vi "W7XBolo2017_Flo.vi"(1 "FPGA VI Reference In":refnum<k20>) -> (0 "FPGA VI Reference Out":refnum<k20>)   [LabVIEW 2014]
uses:
  <vilib>/Platform/TimedLoop/XDataNode/timing_clust.ctl
  <vilib>/Platform/TimedLoop/XDataNode/nitl_modes.ctl
  <vilib>/Platform/TimedLoop/XDataNode/wakeup.ctl
  <vilib>/userdefined/High Color/nirio_resource_hc.ctl
  <vilib>/FPGAPlugInAG/PCI-7813R/niLvFpga_Open_PCI-7813R.vi
  <vilib>/Utility/error.llb/Error Cluster From Error Code.vi
  <vilib>/rvi/errors/niLvFpgaAdjustHostInterfaceError.vi
  <vilib>/Utility/file.llb/Read From Spreadsheet File (I64).vi
  <vilib>/rvi/interface/common/niFpgaWaitOnOcc.vi
  <vilib>/httpClient/POSTBuffer.vi
  <vilib>/FPGAPlugInAG/PCI-7813R/niLvFpga_Close_PCI-7813R.vi
  <vilib>/Platform/TimedLoop/XDataNode/XDataNode.xnode
  <vilib>/rvi/interface/nirviOpenFPGA/nirviOpenFPGA.xnode
  FPGA Bitfiles/W7XBolo2017_FPGATarget_FlorianDefault.lvbitx
  f_main_2014.vi
  <vilib>/rvi/interface/nirviReadWriteControl/nirviReadWriteControl.xnode
  <vilib>/rvi/interface/nirviMethod/nirviMethod.xnode
  <vilib>/rvi/interface/nirviCloseFPGA/nirviCloseFPGA.xnode
  <vilib>/Platform/TimedLoop/XDataNode/XDNodeRunTimeDep.lvlib
  <vilib>/Analysis/NI_AALBase.lvlib
  <vilib>/httpClient/LabVIEWHTTPClient.lvlib
  NiFpgaLv.dll
  <vilib>/FPGAPlugInAG/PCI-7813R/niLvFpga_AcknowledgeIrq_PCI-7813R.vi
  <vilib>/FPGAPlugInAG/PCI-7813R/niLvFpga_ConfigureFifo_PCI-7813R.vi
  <vilib>/rvi/errors/niLvFpgaMergeErrorWithErrorCode.vi
panel:
  out "DAQ Timer":dbl
  in  "chanDescs":T1(array[cluster])=[{"name"="HBCm_U30_01", "active"=1, "physicalQuantity"={"type"="A"}}, {"name"="HBCm_U30_02", "active"=1, "physicalQuantity"={"type"="A"}}, {"name"="HBCm_U30_03", "active"=1, "physicalQuantity"={"type"="A"}}, {"name"="HBCm_U30_04", "active"=1, "physicalQuantity"={"type"="A"}}, {"name"="HBCm_U30_05", "active"=1, "physicalQuantity"={"type"="A"}}, {"name"="HBCm_U30_06", "active"=1, "physicalQuantity"={"type"="A"}}, {"name"="HBCm_U30_07", "active"=1, "physicalQuantity"={"type"="A"}}, {"name"="HBCm_U30_08", "active"=1, "physicalQuantity"={"type"="A"}}, {"name"="HBCm_U30_09", "active"=1, "physicalQuantity"={"type"="A"}}, {"name"="HBCm_U30_10", "active"=1, "physicalQuantity"={"type"="A"}}, {"name"="HBCm_U30_11", "active"=1, "physicalQuantity"={"type"="A"}}, {"name"="HBCm_U30_12", "active"=1, "physicalQuantity"={"type"="A"}}, {"name"="HBCm_U30_013", "active"=1, "physicalQuantity"={"type"="A"}}, {"name"="HBCm_U30_14", "active"=1, "physicalQuantity"={"type"="A"}}, {"name"="HBCm_U30_15", "active"=1, "physicalQuantity"={"type"="A"}}, {"name"="HBCm_U30_16", "active"=1, "physicalQuantity"={"type"="A"}}, {"name"="HBCm_U30_17", "active"=1, "physicalQuantity"={"type"="A"}}, {"name"="HBCm_U30_18", "active"=1, "physicalQuantity"={"type"="A"}}, {"name"="HBCm_U30_19", "active"=1, "physicalQuantity"={"type"="A"}}, {"name"="HBCm_U30_20", "active"=1, "physicalQuantity"={"type"="A"}}, {"name"="HBCm_U30_21", "active"=1, "physicalQuantity"={"type"="A"}}, {"name"="HBCm_U30_22", "active"=1, "physicalQuantity"={"type"="A"}}, {"name"="HBCm_U30_23", "active"=1, "physicalQuantity"={"type"="A"}}, {"name"="HBCm_U30_24", "active"=1, "physicalQuantity"={"type"="A"}}, {"name"="HBCm_U30_25", "active"=1, "physicalQuantity"={"type"="A"}}, {"name"="HBCm_U30_26", "active"=1, "physicalQuantity"={"type"="A"}}, {"name"="HBCm_U30_27", "active"=1, "physicalQuantity"={"type"="A"}}, {"name"="HBCm_U30_28", "active"=1, "physicalQuantity"={"type"="A"}}, {"name"="HBCm_U30_29", "active"=1, "physicalQuantity"={"type"="A"}}, {"name"="HBCm_U30_30", "active"=1, "physicalQuantity"={"type"="A"}}, {"name"="HBCm_U30_31", "active"=1, "physicalQuantity"={"type"="A"}}, {"name"="HBCm_U30_32", "active"=1, "physicalQuantity"={"type"="A"}}, {"name"="VBCm_V21_01", "active"=1, "physicalQuantity"={"type"="A"}}, {"name"="VBCm_V21_02", "active"=1, "physicalQuantity"={"type"="A"}}, {"name"="VBCm_V21_03", "active"=1, "physicalQuantity"={"type"="A"}}, {"name"="VBCm_V21_04", "active"=1, "physicalQuantity"={"type"="A"}}, {"name"="VBCm_V21_05", "active"=1, "physicalQuantity"={"type"="A"}}, {"name"="VBCm_V21_06", "active"=1, "physicalQuantity"={"type"="A"}}, {"name"="VBCm_V21_07", "active"=1, "physicalQuantity"={"type"="A"}}, {"name"="VBCm_V21_08", "active"=1, "physicalQuantity"={"type"="A"}}, {"name"="VBCm_V21_09", "active"=1, "physicalQuantity"={"type"="A"}}, {"name"="VBCm_V21_10", "active"=1, "physicalQuantity"={"type"="A"}}, {"name"="VBCm_V21_11", "active"=1, "physicalQuantity"={"type"="A"}}, {"name"="VBCm_V21_12", "active"=1, "physicalQuantity"={"type"="A"}}, {"name"="VBCm_V21_13", "active"=1, "physicalQuantity"={"type"="A"}}, {"name"="VBCm_V21_14", "active"=1, "physicalQuantity"={"type"="A"}}, {"name"="VBCm_V21_15", "active"=1, "physicalQuantity"={"type"="A"}}, {"name"="VBCm_V21_16", "active"=1, "physicalQuantity"={"type"="A"}}, {"name"="VBCm_V21_17", "active"=1, "physicalQuantity"={"type"="A"}}, {"name"="VBCm_V21_18", "active"=1, "physicalQuantity"={"type"="A"}}, {"name"="VBCm_V21_19", "active"=1, "physicalQuantity"={"type"="A"}}, {"name"="VBCm_V21_20", "active"=1, "physicalQuantity"={"type"="A"}}, {"name"="VBCm_V21_21", "active"=1, "physicalQuantity"={"type"="A"}}, {"name"="VBCm_V21_22", "active"=1, "physicalQuantity"={"type"="A"}}, {"name"="VBCm_V21_23", "active"=1, "physicalQuantity"={"type"="A"}}, {"name"="VBCm_V21_24", "active"=1, "physicalQuantity"={"type"="A"}}, {"name"="VBCm_V21_25", "active"=1, "physicalQuantity"={"type"="A"}}, {"name"="VBCm_V21_26", "active"=1, "physicalQuantity"={"type"="A"}}, {"name"="VBCm_V21_27", "active"=1, "physicalQuantity"={"type"="A"}}, {"name"="VBCm_V21_28", "active"=1, "physicalQuantity"={"type"="A"}}, {"name"="VBCm_V21_29", "active"=1, "physicalQuantity"={"type"="A"}}, {"name"="VBCm_V21_30", "active"=1, "physicalQuantity"={"type"="A"}}, {"name"="VBCm_V21_31", "active"=1, "physicalQuantity"={"type"="A"}}, {"name"="VBCm_V21_32", "active"=1, "physicalQuantity"={"type"="A"}}, {"name"="VBCm_V21_33", "active"=1, "physicalQuantity"={"type"="A"}}, {"name"="VBCm_V21_34", "active"=1, "physicalQuantity"={"type"="A"}}, {"name"="VBCm_V21_35", "active"=1, "physicalQuantity"={"type"="A"}}, {"name"="VBCm_V21_36", "active"=1, "physicalQuantity"={"type"="A"}}, {"name"="VBCm_V21_37", "active"=1, "physicalQuantity"={"type"="A"}}, {"name"="VBCm_V21_38", "active"=1, "physicalQuantity"={"type"="A"}}, {"name"="VBCm_V21_39", "active"=1, "physicalQuantity"={"type"="A"}}, {"name"="VBCm_V21_40", "active"=1, "physicalQuantity"={"type"="A"}}, {"name"="VBCs_V21_01", "active"=1, "physicalQuantity"={"type"="A"}}, {"name"="VBCs_V21_02", "active"=1, "physicalQuantity"={"type"="A"}}, {"name"="VBCs_V21_03", "active"=1, "physicalQuantity"={"type"="A"}}, {"name"="VBCs_V21_04", "active"=1, "physicalQuantity"={"type"="A"}}, {"name"="VBCs_V21_05", "active"=1, "physicalQuantity"={"type"="A"}}, {"name"="VBCs_V21_06", "active"=1, "physicalQuantity"={"type"="A"}}, {"name"="VBCs_V21_07", "active"=1, "physicalQuantity"={"type"="A"}}, {"name"="VBCs_V21_08", "active"=1, "physicalQuantity"={"type"="A"}}, {"name"="HBCs_U30_01", "active"=1, "physicalQuantity"={"type"="A"}}, {"name"="HBCs_U30_02", "active"=1, "physicalQuantity"={"type"="A"}}, {"name"="HBCs_U30_03", "active"=1, "physicalQuantity"={"type"="A"}}, {"name"="HBCs_U30_04", "active"=1, "physicalQuantity"={"type"="A"}}, {"name"="HBCs_U30_05", "active"=1, "physicalQuantity"={"type"="A"}}, {"name"="HBCs_U30_06", "active"=1, "physicalQuantity"={"type"="A"}}, {"name"="HBCs_U30_07", "active"=1, "physicalQuantity"={"type"="A"}}, {"name"="HBCs_U30_08", "active"=1, "physicalQuantity"={"type"="A"}}, {"name"="HBCs_U30_09", "active"=1, "physicalQuantity"={"type"="A"}}, {"name"="HBCs_U30_10", "active"=1, "physicalQuantity"={"type"="A"}}, {"name"="HBCs_U30_11", "active"=1, "physicalQuantity"={"type"="A"}}, {"name"="HBCs_U30_12", "active"=1, "physicalQuantity"={"type"="A"}}, {"name"="HBCs_U30_13", "active"=1, "physicalQuantity"={"type"="A"}}, {"name"="HBCs_U30_14", "active"=1, "physicalQuantity"={"type"="A"}}, {"name"="HBCs_U30_15", "active"=1, "physicalQuantity"={"type"="A"}}, {"name"="HBCs_U30_16", "active"=1, "physicalQuantity"={"type"="A"}}]
  in  "Tab Control 7":T2(tab)
  in  "FreqSelRing":u16(ring) items=["0.8 ms", "1.6 ms", "3.2 ms", "6.4 ms", "12.8 ms", "19.2 ms"]
  in  "SecondFilter":bool=TRUE
  out "SampleTime":sgl=0.0004
  in  "Global or Individual\nDAC Settings loaded \nfrom File":bool=TRUE caption="Range?"
  in  "DAC Range Setting":u8(knob)=3 scale=0.0..3.0
  in  "No. of Samples:":u32=10000
  out "Measured Time \nfor DAQ [ms] \nShould ~ correspond to\nSampleTime * Samples":u32=8048
  in  "Trigger Source":i32(slide)=1 scale=0.0..2.0
  in  "Set Manual Time [ns]":i64=1503619200000000000
  out "Presamples \n(If -1, then no trigger detected)":i32
  out "DAQ wait time (should be = TWT":i32=-1
  out "Countdown Time":u32
  out "Calibration Time":u32
  out "Total wait time (TWT)\nTypically 59 s":u32
  in  "Pre-start time (ms) of DAQ \nTypically set to 1000 ms":i32=1000
  out "Fixed T-60sec before T1 = T0":i32=60000
  in  "Wait-Time until Trigger\npublished on CODA\ntypically 10 s":u32=10000
  in  "Tau00":dbl[](array[numeric])
  in  "Kappa00":dbl[](array[numeric])
  in  "RB000":dbl[](array[numeric])
  in  "Switch to fixed \nCalibration Values":bool
  in  "Clear all Values \nfrom Beginning":bool
  in  "Cancel Button":bool
  out "Actual Depth":u32=256
  out "T-Start [for Display)\nShould be -1 [s]":sgl=-1.0
  in  "Trigger No Choice\nfrom MDS+ Website\n0 for old\n1 during OP":i32
  out "body chanDesc":string="Test/raw/W7X/QSB_Bolometry/File_PARLOG/ created."
  out "headers chanDesc":string="HTTP/1.1 201 Created\r\nServer: Apache-Coyote/1.1\r\nLocation: http://archive-webapi.ipp-hgw.mpg.de/Test/raw/W7X/QSB_Bolometry/File_PARLOG/\r\nContent-Type: text/plain\r\nTransfer-Encoding: chunked\r\nDate: Wed, 15 Jul 2015 13:52:20 GMT\r\n\r\n"
  out "parms error out":errorcluster
  in  "Tab Control":T3(tab)
  in  "Tab Control 4":enum32{"1 to 64", "65 to 128"}(tab)
  out "Raw 33-64":T4={"Channels 33 - 40"={"tstart"=-1.0, "FPGSampleTime"=0.0007999999797903001, array8x10000[80000 elements]}, "Channels 41 - 48"={"tstart"=-1.0, "FPGSampleTime"=0.0007999999797903001, array8x10000[80000 elements]}, "Channels 49 - 56"={"tstart"=-1.0, "FPGSampleTime"=0.0007999999797903001, array8x10000[80000 elements]}, "Channels 57 - 64"={"tstart"=-1.0, "FPGSampleTime"=0.0007999999797903001, array8x10000[80000 elements]}}
  out "Raw 1-32":T5={"Channels 1- 8"={"tstart"=-1.0, "FPGSampleTime"=0.0007999999797903001, array8x10000[80000 elements]}, "Channels 9 - 16"={"tstart"=-1.0, "FPGSampleTime"=0.0007999999797903001, array8x10000[80000 elements]}, "Channels 17 - 24"={"tstart"=-1.0, "FPGSampleTime"=0.0007999999797903001, array8x10000[80000 elements]}, "Channels 25 - 32"={"tstart"=-1.0, "FPGSampleTime"=0.0007999999797903001, array8x10000[80000 elements]}}
  out "Raw 97 - 128":T6
  out "Raw 65 - 97":T7={"Channels 65 - 71"={"tstart"=-1.0, "FPGSampleTime"=0.0007999999797903001, array8x10000[80000 elements]}, "Channels 73 - 80"={"tstart"=0.0, "FPGSampleTime"=0.0, []}, "Channels 81 - 88"={"tstart"=0.0, "FPGSampleTime"=0.0, []}, "Channels 89- 96"={"tstart"=0.0, "FPGSampleTime"=0.0, []}}
  in  "Tab Control 6":enum32{"1 to 64", "65 to 128"}(tab)=enum."65 to 128"
  out "Pow 33-64":T4
  out "Pow 1-32":T5={"Channels 1- 8"={"tstart"=-1.0, "FPGSampleTime"=0.0007999999797903001, array8x10000[80000 elements]}, "Channels 9 - 16"={"tstart"=-1.0, "FPGSampleTime"=0.0007999999797903001, array8x10000[80000 elements]}, "Channels 17 - 24"={"tstart"=0.0, "FPGSampleTime"=0.0, []}, "Channels 25 - 32"={"tstart"=0.0, "FPGSampleTime"=0.0, []}}
  out "Pow 97 - 128":T6
  out "Pow 65 - 96":T7={"Channels 65 - 71"={"tstart"=-1.0, "FPGSampleTime"=0.0007999999797903001, array8x10000[80000 elements]}, "Channels 73 - 80"={"tstart"=0.0, "FPGSampleTime"=0.0, []}, "Channels 81 - 88"={"tstart"=0.0, "FPGSampleTime"=0.0, []}, "Channels 89- 96"={"tstart"=0.0, "FPGSampleTime"=0.0, []}}
  out "RangeIndex":u8[](array[numeric])
  out "DACbits 2":u16[](array[numeric])
  in  "file path (dialog if empty)":path=path "C:/W7-X-DAQ-Data/_DAQ_Ranges.txt"
  in  "Tab Control 2":T8(tab)
  out "Offset 1-32":T5
  out "Offset 33-64":T4
  out "Offset 65 - 96":T7
  out "Offset 97 - 128":T6
  out "Mean (mV)":dbl[](array[numeric]) format="%10.6f"
  out "Peak to Peak \n      (microV)":dbl[](array[numeric]) format="%10.6f"
  out "StandardDeviation\n        (microV)":dbl[](array[numeric]) format="%10.7f"
  out "RefStatus 65-96":bool[](array[boolean])
  out "RefStatus 33-64":bool[](array[boolean])
  out "RefStatus 1-32":bool[](array[boolean])
  out "RefStatus 97-128":bool[](array[boolean])
  out "MessStatus 1-32":bool[](array[boolean])
  out "MessStatus 33-64":bool[](array[boolean])
  out "MessStatus 97-128":bool[](array[boolean])
  out "MessStatus 65-96":bool[](array[boolean])
  in  "Tab Control 5":T9(tab)
  out "MessCal 17-32":T10
  out "MessCal 1-16":T11
  out "MessCal 49 - 64":T12
  out "MessCal 33 - 49":T13
  out "MessCal 81 - 96":T14
  out "MessCal 65 - 80":T15
  out "MessCal 113 - 128":T16
  out "MessCal 97 - 112":T17
  out "RMESS":dbl[](array[numeric])
  out "KappaM":dbl[](array[numeric]) format="%10.4e"
  out "TauM":dbl[](array[numeric]) format="%10.4f"
  in  "Tab Control 3":T9(tab)=enum."97 to 128"
  out "RefCal 17-32":T10
  out "RefCal 1-16":T11
  out "RefCal 49 - 64":T12
  out "RefCal 33 - 48":T13
  out "RefCal 65 - 80":T15
  out "RefCal 81 - 96":T14
  out "RefCal 113 - 128":T16
  out "RefCal 97 - 112":T17
  out "TauR":dbl[](array[numeric]) caption="TauM" format="%10.4f"
  out "KappaR":dbl[](array[numeric]) format="%10.4e"
  out "RREF":dbl[](array[numeric])
  out "Parlog error out":errorcluster
  out "Parlog error out  2":errorcluster
  out "Parlog error out  3":errorcluster
  out "error out":errorcluster
  out "Timed Out 2":bool
  out "Fehler":bool
  out "Fehler READ U+P":bool
  out "FilterTimeOut":bool
  out "result":bool
  out "chanDescs 2":T1(array[cluster])=[{"name"="HBCm_U30_01", "active"=1, "physicalQuantity"={"type"="A"}}, {"name"="HBCm_U30_02", "active"=1, "physicalQuantity"={"type"="A"}}, {"name"="HBCm_U30_03", "active"=1, "physicalQuantity"={"type"="A"}}, {"name"="HBCm_U30_04", "active"=1, "physicalQuantity"={"type"="A"}}, {"name"="HBCm_U30_05", "active"=1, "physicalQuantity"={"type"="A"}}, {"name"="HBCm_U30_06", "active"=1, "physicalQuantity"={"type"="A"}}, {"name"="HBCm_U30_07", "active"=1, "physicalQuantity"={"type"="A"}}, {"name"="HBCm_U30_08", "active"=1, "physicalQuantity"={"type"="A"}}, {"name"="HBCm_U30_09", "active"=1, "physicalQuantity"={"type"="A"}}, {"name"="HBCm_U30_10", "active"=1, "physicalQuantity"={"type"="A"}}, {"name"="HBCm_U30_11", "active"=1, "physicalQuantity"={"type"="A"}}, {"name"="HBCm_U30_12", "active"=1, "physicalQuantity"={"type"="A"}}, {"name"="HBCm_U30_13", "active"=1, "physicalQuantity"={"type"="A"}}, {"name"="HBCm_U30_14", "active"=1, "physicalQuantity"={"type"="A"}}, {"name"="HBCm_U30_15", "active"=1, "physicalQuantity"={"type"="A"}}, {"name"="HBCm_U30_16", "active"=1, "physicalQuantity"={"type"="A"}}, {"name"="HBCm_U30_17", "active"=1, "physicalQuantity"={"type"="A"}}, {"name"="HBCm_U30_18", "active"=1, "physicalQuantity"={"type"="A"}}, {"name"="HBCm_U30_19", "active"=1, "physicalQuantity"={"type"="A"}}, {"name"="HBCm_U30_20", "active"=1, "physicalQuantity"={"type"="A"}}, {"name"="HBCm_U30_21", "active"=1, "physicalQuantity"={"type"="A"}}, {"name"="HBCm_U30_22", "active"=1, "physicalQuantity"={"type"="A"}}, {"name"="HBCm_U30_23", "active"=1, "physicalQuantity"={"type"="A"}}, {"name"="HBCm_U30_24", "active"=1, "physicalQuantity"={"type"="A"}}, {"name"="HBCm_U30_25", "active"=1, "physicalQuantity"={"type"="A"}}, {"name"="HBCm_U30_26", "active"=1, "physicalQuantity"={"type"="A"}}, {"name"="HBCm_U30_27", "active"=1, "physicalQuantity"={"type"="A"}}, {"name"="HBCm_U30_28", "active"=1, "physicalQuantity"={"type"="A"}}, {"name"="HBCm_U30_29", "active"=1, "physicalQuantity"={"type"="A"}}, {"name"="HBCm_U30_30", "active"=1, "physicalQuantity"={"type"="A"}}, {"name"="HBCm_U30_31", "active"=1, "physicalQuantity"={"type"="A"}}, {"name"="HBCm_U30_32", "active"=1, "physicalQuantity"={"type"="A"}}, {"name"="VBCm_V21_01", "active"=1, "physicalQuantity"={"type"="A"}}, {"name"="VBCm_V21_02", "active"=1, "physicalQuantity"={"type"="A"}}, {"name"="VBCm_V21_03", "active"=1, "physicalQuantity"={"type"="A"}}, {"name"="VBCm_V21_04", "active"=1, "physicalQuantity"={"type"="A"}}, {"name"="VBCm_V21_05", "active"=1, "physicalQuantity"={"type"="A"}}, {"name"="VBCm_V21_06", "active"=1, "physicalQuantity"={"type"="A"}}, {"name"="VBCm_V21_07", "active"=1, "physicalQuantity"={"type"="A"}}, {"name"="VBCm_V21_08", "active"=1, "physicalQuantity"={"type"="A"}}, {"name"="VBCm_V21_09", "active"=1, "physicalQuantity"={"type"="A"}}, {"name"="VBCm_V21_10", "active"=1, "physicalQuantity"={"type"="A"}}, {"name"="VBCm_V21_11", "active"=1, "physicalQuantity"={"type"="A"}}, {"name"="VBCm_V21_12", "active"=1, "physicalQuantity"={"type"="A"}}, {"name"="VBCm_V21_13", "active"=1, "physicalQuantity"={"type"="A"}}, {"name"="VBCm_V21_14", "active"=1, "physicalQuantity"={"type"="A"}}, {"name"="VBCm_V21_15", "active"=1, "physicalQuantity"={"type"="A"}}, {"name"="VBCm_V21_16", "active"=1, "physicalQuantity"={"type"="A"}}, {"name"="VBCm_V21_17", "active"=1, "physicalQuantity"={"type"="A"}}, {"name"="VBCm_V21_18", "active"=1, "physicalQuantity"={"type"="A"}}, {"name"="VBCm_V21_19", "active"=1, "physicalQuantity"={"type"="A"}}, {"name"="VBCm_V21_20", "active"=1, "physicalQuantity"={"type"="A"}}, {"name"="VBCm_V21_21", "active"=1, "physicalQuantity"={"type"="A"}}, {"name"="VBCm_V21_22", "active"=1, "physicalQuantity"={"type"="A"}}, {"name"="VBCm_V21_23", "active"=1, "physicalQuantity"={"type"="A"}}, {"name"="VBCm_V21_24", "active"=1, "physicalQuantity"={"type"="A"}}, {"name"="VBCm_V21_25", "active"=1, "physicalQuantity"={"type"="A"}}, {"name"="VBCm_V21_26", "active"=1, "physicalQuantity"={"type"="A"}}, {"name"="VBCm_V21_27", "active"=1, "physicalQuantity"={"type"="A"}}, {"name"="VBCm_V21_28", "active"=1, "physicalQuantity"={"type"="A"}}, {"name"="VBCm_V21_29", "active"=1, "physicalQuantity"={"type"="A"}}, {"name"="VBCm_V21_30", "active"=1, "physicalQuantity"={"type"="A"}}, {"name"="VBCm_V21_31", "active"=1, "physicalQuantity"={"type"="A"}}, {"name"="VBCm_V21_32", "active"=1, "physicalQuantity"={"type"="A"}}, {"name"="VBCm_V21_33", "active"=1, "physicalQuantity"={"type"="A"}}, {"name"="VBCm_V21_34", "active"=1, "physicalQuantity"={"type"="A"}}, {"name"="VBCm_V21_35", "active"=1, "physicalQuantity"={"type"="A"}}, {"name"="VBCm_V21_36", "active"=1, "physicalQuantity"={"type"="A"}}, {"name"="VBCm_V21_37", "active"=1, "physicalQuantity"={"type"="A"}}, {"name"="VBCm_V21_38", "active"=1, "physicalQuantity"={"type"="A"}}, {"name"="VBCm_V21_39", "active"=1, "physicalQuantity"={"type"="A"}}, {"name"="VBCm_V21_40", "active"=1, "physicalQuantity"={"type"="A"}}, {"name"="VBCs_V21_01", "active"=1, "physicalQuantity"={"type"="A"}}, {"name"="VBCs_V21_02", "active"=1, "physicalQuantity"={"type"="A"}}, {"name"="VBCs_V21_03", "active"=1, "physicalQuantity"={"type"="A"}}, {"name"="VBCs_V21_04", "active"=1, "physicalQuantity"={"type"="A"}}, {"name"="VBCs_V21_05", "active"=1, "physicalQuantity"={"type"="A"}}, {"name"="VBCs_V21_06", "active"=1, "physicalQuantity"={"type"="A"}}, {"name"="VBCs_V21_07", "active"=1, "physicalQuantity"={"type"="A"}}, {"name"="VBCs_V21_08", "active"=1, "physicalQuantity"={"type"="A"}}, {"name"="HBCs_U30_01", "active"=1, "physicalQuantity"={"type"="A"}}, {"name"="HBCs_U30_02", "active"=1, "physicalQuantity"={"type"="A"}}, {"name"="HBCs_U30_03", "active"=1, "physicalQuantity"={"type"="A"}}, {"name"="HBCs_U30_04", "active"=1, "physicalQuantity"={"type"="A"}}, {"name"="HBCs_U30_05", "active"=1, "physicalQuantity"={"type"="A"}}, {"name"="HBCs_U30_06", "active"=1, "physicalQuantity"={"type"="A"}}, {"name"="HBCs_U30_07", "active"=1, "physicalQuantity"={"type"="A"}}, {"name"="HBCs_U30_08", "active"=1, "physicalQuantity"={"type"="A"}}, {"name"="HBCs_U30_09", "active"=1, "physicalQuantity"={"type"="A"}}, {"name"="HBCs_U30_10", "active"=1, "physicalQuantity"={"type"="A"}}, {"name"="HBCs_U30_11", "active"=1, "physicalQuantity"={"type"="A"}}, {"name"="HBCs_U30_12", "active"=1, "physicalQuantity"={"type"="A"}}, {"name"="HBCs_U30_13", "active"=1, "physicalQuantity"={"type"="A"}}, {"name"="HBCs_U30_14", "active"=1, "physicalQuantity"={"type"="A"}}, {"name"="HBCs_U30_15", "active"=1, "physicalQuantity"={"type"="A"}}, {"name"="HBCs_U30_16", "active"=1, "physicalQuantity"={"type"="A"}}, {"name"="Test96", "active"=1, "physicalQuantity"={"type"="A"}}, {"name"="Test97", "active"=0, "physicalQuantity"={"type"=""}}]
  out "error out Cal":errorcluster
  in  "stop":bool
  out "Acquired Samples:":u32(slide) scale=-1.0..10000.0
  out "state":string="Wait for Start"
  # "Largest Offset ~ 20 mV\n40 mV Range should work \nfor all channels"
  # "Sample Rate Settings"
  # "FilterSelection"
  # "Set manual time above"
  # "Get last trigger fr om \nhttp://sv-coda-wsvc-3/last_trigger"
  # "Get UTC Time not working"
  # "WENDELSTEIN - 7-X Bolometer DAQ System"
  # "ver 2017"
  # "If individual Range DAC Setting is selected, \nthe gain Range is loaded from following file:"
  # "DAC Range shown for check:"
types:
  T1 = cluster{"name":string, "active":i32, "physicalQuantity":cluster{"type":string}}[]
  T2 = enum32{"DAQ Settings", "Trigger Selection", "Fixed Calib Values", "Experimental"}
  T3 = enum32{"Raw", "Power", "Indiviudal Range Settings", "Offsets", "Status", "CalibMess", "CalibRef", "Errors and others"}
  T4 = cluster{"Channels 33 - 40":cluster{"tstart":dbl, "FPGSampleTime":dbl, dbl[][]}, "Channels 41 - 48":cluster{"tstart":dbl, "FPGSampleTime":dbl, dbl[][]}, "Channels 49 - 56":cluster{"tstart":dbl, "FPGSampleTime":dbl, dbl[][]}, "Channels 57 - 64":cluster{"tstart":dbl, "FPGSampleTime":dbl, dbl[][]}}
  T5 = cluster{"Channels 1- 8":cluster{"tstart":dbl, "FPGSampleTime":dbl, dbl[][]}, "Channels 9 - 16":cluster{"tstart":dbl, "FPGSampleTime":dbl, dbl[][]}, "Channels 17 - 24":cluster{"tstart":dbl, "FPGSampleTime":dbl, dbl[][]}, "Channels 25 - 32":cluster{"tstart":dbl, "FPGSampleTime":dbl, dbl[][]}}
  T6 = cluster{"Channels 97 - 104":cluster{"tstart":dbl, "FPGSampleTime":dbl, dbl[][]}, "Channels 105 - 112":cluster{"tstart":dbl, "FPGSampleTime":dbl, dbl[][]}, "Channels 113 - 120":cluster{"tstart":dbl, "FPGSampleTime":dbl, dbl[][]}, "Channels 121 - 128":cluster{"tstart":dbl, "FPGSampleTime":dbl, dbl[][]}}
  T7 = cluster{"Channels 65 - 71":cluster{"tstart":dbl, "FPGSampleTime":dbl, dbl[][]}, "Channels 73 - 80":cluster{"tstart":dbl, "FPGSampleTime":dbl, dbl[][]}, "Channels 81 - 88":cluster{"tstart":dbl, "FPGSampleTime":dbl, dbl[][]}, "Channels 89- 96":cluster{"tstart":dbl, "FPGSampleTime":dbl, dbl[][]}}
  T8 = enum32{"1 to 32", "33 to 64", "65 to 96", "97 to128"}
  T9 = enum32{"1 to 32", "33 to 64", "65 to 96", "97 to 128"}
  T10 = cluster{"Channels 17 - 20":cluster{"tstart":sgl, "dt":sgl, "OutArray":dbl[][]}, "Channels 21 - 24":cluster{"tstart":sgl, "dt":sgl, "OutArray":dbl[][]}, "Channels 25 - 28":cluster{"tstart":sgl, "dt":sgl, "OutArray":dbl[][]}, "Channels 29 - 32":cluster{"tstart":sgl, "dt":sgl, "OutArray":dbl[][]}}
  T11 = cluster{"Channels 1- 4":cluster{"tstart":sgl, "dt":sgl, "OutArray":dbl[][]}, "Channels 5 - 8":cluster{"tstart":sgl, "dt":sgl, "OutArray":dbl[][]}, "Channels 9 - 12":cluster{"tstart":sgl, "dt":sgl, "OutArray":dbl[][]}, "Channels 13 - 16":cluster{"tstart":sgl, "dt":sgl, "OutArray":dbl[][]}}
  T12 = cluster{"Channels 49 - 52":cluster{"tstart":sgl, "dt":sgl, "OutArray":dbl[][]}, "Channels 53 - 56":cluster{"tstart":sgl, "dt":sgl, "OutArray":dbl[][]}, "Channels 57 - 60":cluster{"tstart":sgl, "dt":sgl, "OutArray":dbl[][]}, "Channels 61 - 64":cluster{"tstart":sgl, "dt":sgl, "OutArray":dbl[][]}}
  T13 = cluster{"Channels 33 - 36":cluster{"tstart":sgl, "dt":sgl, "OutArray":dbl[][]}, "Channels 37 - 40":cluster{"tstart":sgl, "dt":sgl, "OutArray":dbl[][]}, "Channels 41 - 44":cluster{"tstart":sgl, "dt":sgl, "OutArray":dbl[][]}, "Channels 45 - 48":cluster{"tstart":sgl, "dt":sgl, "OutArray":dbl[][]}}
  T14 = cluster{"Channels 81 - 84":cluster{"tstart":sgl, "dt":sgl, "OutArray":dbl[][]}, "Channels 85 - 88":cluster{"tstart":sgl, "dt":sgl, "OutArray":dbl[][]}, "Channels 89 - 92":cluster{"tstart":sgl, "dt":sgl, "OutArray":dbl[][]}, "Channels 93 - 96":cluster{"tstart":sgl, "dt":sgl, "OutArray":dbl[][]}}
  T15 = cluster{"Channels 65 - 68":cluster{"tstart":sgl, "dt":sgl, "OutArray":dbl[][]}, "Channels 69 - 72":cluster{"tstart":sgl, "dt":sgl, "OutArray":dbl[][]}, "Channels 73 - 76":cluster{"tstart":sgl, "dt":sgl, "OutArray":dbl[][]}, "Channels 77 - 80":cluster{"tstart":sgl, "dt":sgl, "OutArray":dbl[][]}}
  T16 = cluster{"Channels 113 - 116":cluster{"tstart":sgl, "dt":sgl, "OutArray":dbl[][]}, "Channels 117 - 120":cluster{"tstart":sgl, "dt":sgl, "OutArray":dbl[][]}, "Channels 121 - 124":cluster{"tstart":sgl, "dt":sgl, "OutArray":dbl[][]}, "Channels 125 - 128":cluster{"tstart":sgl, "dt":sgl, "OutArray":dbl[][]}}
  T17 = cluster{"Channels 97 - 100":cluster{"tstart":sgl, "dt":sgl, "OutArray":dbl[][]}, "Channels 101 - 104":cluster{"tstart":sgl, "dt":sgl, "OutArray":dbl[][]}, "Channels 104 - 108":cluster{"tstart":sgl, "dt":sgl, "OutArray":dbl[][]}, "Channels 109 - 112":cluster{"tstart":sgl, "dt":sgl, "OutArray":dbl[][]}}
  T18 = cluster{"Nchannel":i16, "ADCbits":i16, "BridgeVoltage (V)":sgl, "ExptSampleFrequency (Hz)":sgl, "CalibSampleFrequency (Hz)":sgl, "CalStep1 (V)":string, "CalStep2 (V)":string, "detector":string}[]
  T19 = cluster{"chanDescs":cluster{"name":string, "active":i32}[]}[]
  T20 = cluster{"tstart":sgl, "dt":sgl, "OutArray":dbl[][]}
  T21 = cluster{"Channels 9 - 12":cluster{"tstart":sgl, "dt":sgl, "OutArray":dbl[][]}, "Channels 9 - 12":cluster{"tstart":sgl, "dt":sgl, "OutArray":dbl[][]}, "Channels 9 - 12":cluster{"tstart":sgl, "dt":sgl, "OutArray":dbl[][]}, "Channels 9 - 12":cluster{"tstart":sgl, "dt":sgl, "OutArray":dbl[][]}}
  T22 = typedef "nirio_resource_hc.ctl" = tag
  T23 = typedef "XDNodeRunTimeDep.lvlib/timing_clust.ctl" = cluster{"Expected End [f-1]":u64, "Actual End [f-1]":u64, "Finished Late? [f-1]":bool, "Expected End [i-1]":u64, "Actual End [i-1]":u64, "Finished Late? [i-1]":bool, "Expected Start [i]":u64, "Actual Start [i]":u64, "Expected Start [f]":u64, "Actual Start [f]":u64, "Source Name":string, "Structure Name":string, "Period":i64, "Deadline":i64, "Offset":i64, "Start":i64, "Priority":i32, "Timeout":i32, "Mode":T24, "Wakeup Reason":T25, "Error":errorcluster, "Source Type":string, "Secondary Source Type":string, "Global End Time":u64, "Global Start Time":u64, "Frame Duration":u64, "Iteration Duration":u64, "Assigned CPU":i32, "I/O Scan Engine Mode":u32}
  T24 = typedef "XDNodeRunTimeDep.lvlib/nitl_modes.ctl" = enum32{"No Change", "Process missed periods, maintain original phase", "Discard missed periods, maintain original phase", "Process missed periods, ignore original phase", "Discard missed periods, ignore original phase"}
  T25 = typedef "XDNodeRunTimeDep.lvlib/wakeup.ctl" = enum32{"Normal", "Aborted", "Asynchronous wakeup", "Timing source error", "Timed loop error", "Timeout"}
  T26 = cluster{"Channels 33 - 40":cluster{"tstart":dbl, "FPGSampleTime":dbl, dbl[][]}, "Channels 41 - 48":cluster{"tstart":dbl, "FPGSampleTime":dbl, dbl[][]}, "Channels 49 - 56":cluster{"tstart":dbl, "FPGSampleTime":dbl, dbl[][]}, "Channels 57 - 58":cluster{"tstart":dbl, "FPGSampleTime":dbl, dbl[][]}}
  T27 = cluster{"Channels 1- 8":cluster{"tstart":sgl, "dt":sgl, "OutArray":dbl[][]}, "Channels 9 - 16":cluster{"tstart":sgl, "dt":sgl, "OutArray":dbl[][]}, "Channels 17 - 24":cluster{"tstart":sgl, "dt":sgl, "OutArray":dbl[][]}, "Channels 25 - 32":cluster{"tstart":sgl, "dt":sgl, "OutArray":dbl[][]}}
  T28 = cluster{"Channels 33 - 40":cluster{"tstart":sgl, "dt":sgl, "OutArray":dbl[][]}, "Channels 41 - 48":cluster{"tstart":sgl, "dt":sgl, "OutArray":dbl[][]}, "Channels 49 - 56":cluster{"tstart":sgl, "dt":sgl, "OutArray":dbl[][]}, "Channels 57 - 58":cluster{"tstart":sgl, "dt":sgl, "OutArray":dbl[][]}}
  T29 = typedef "LabVIEWHTTPClient.lvlib/ClientHandle.ctl" = refnum<k1>
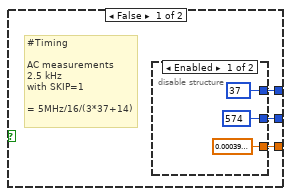
[diagram p5: hidden frame]
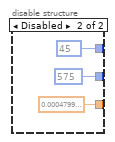
[diagram p6: hidden frame]
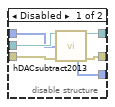
[diagram p7: hidden frame]
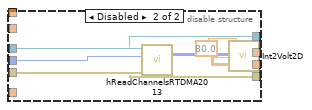
[diagram p8: hidden frame]
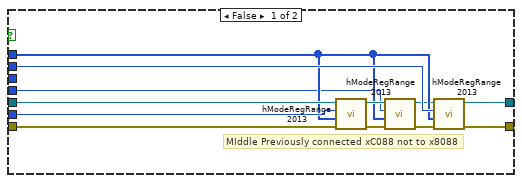
[diagram p9: hidden frame]
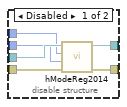
[diagram p10: hidden frame]
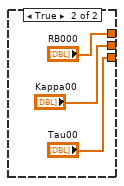
[diagram p11: hidden frame]
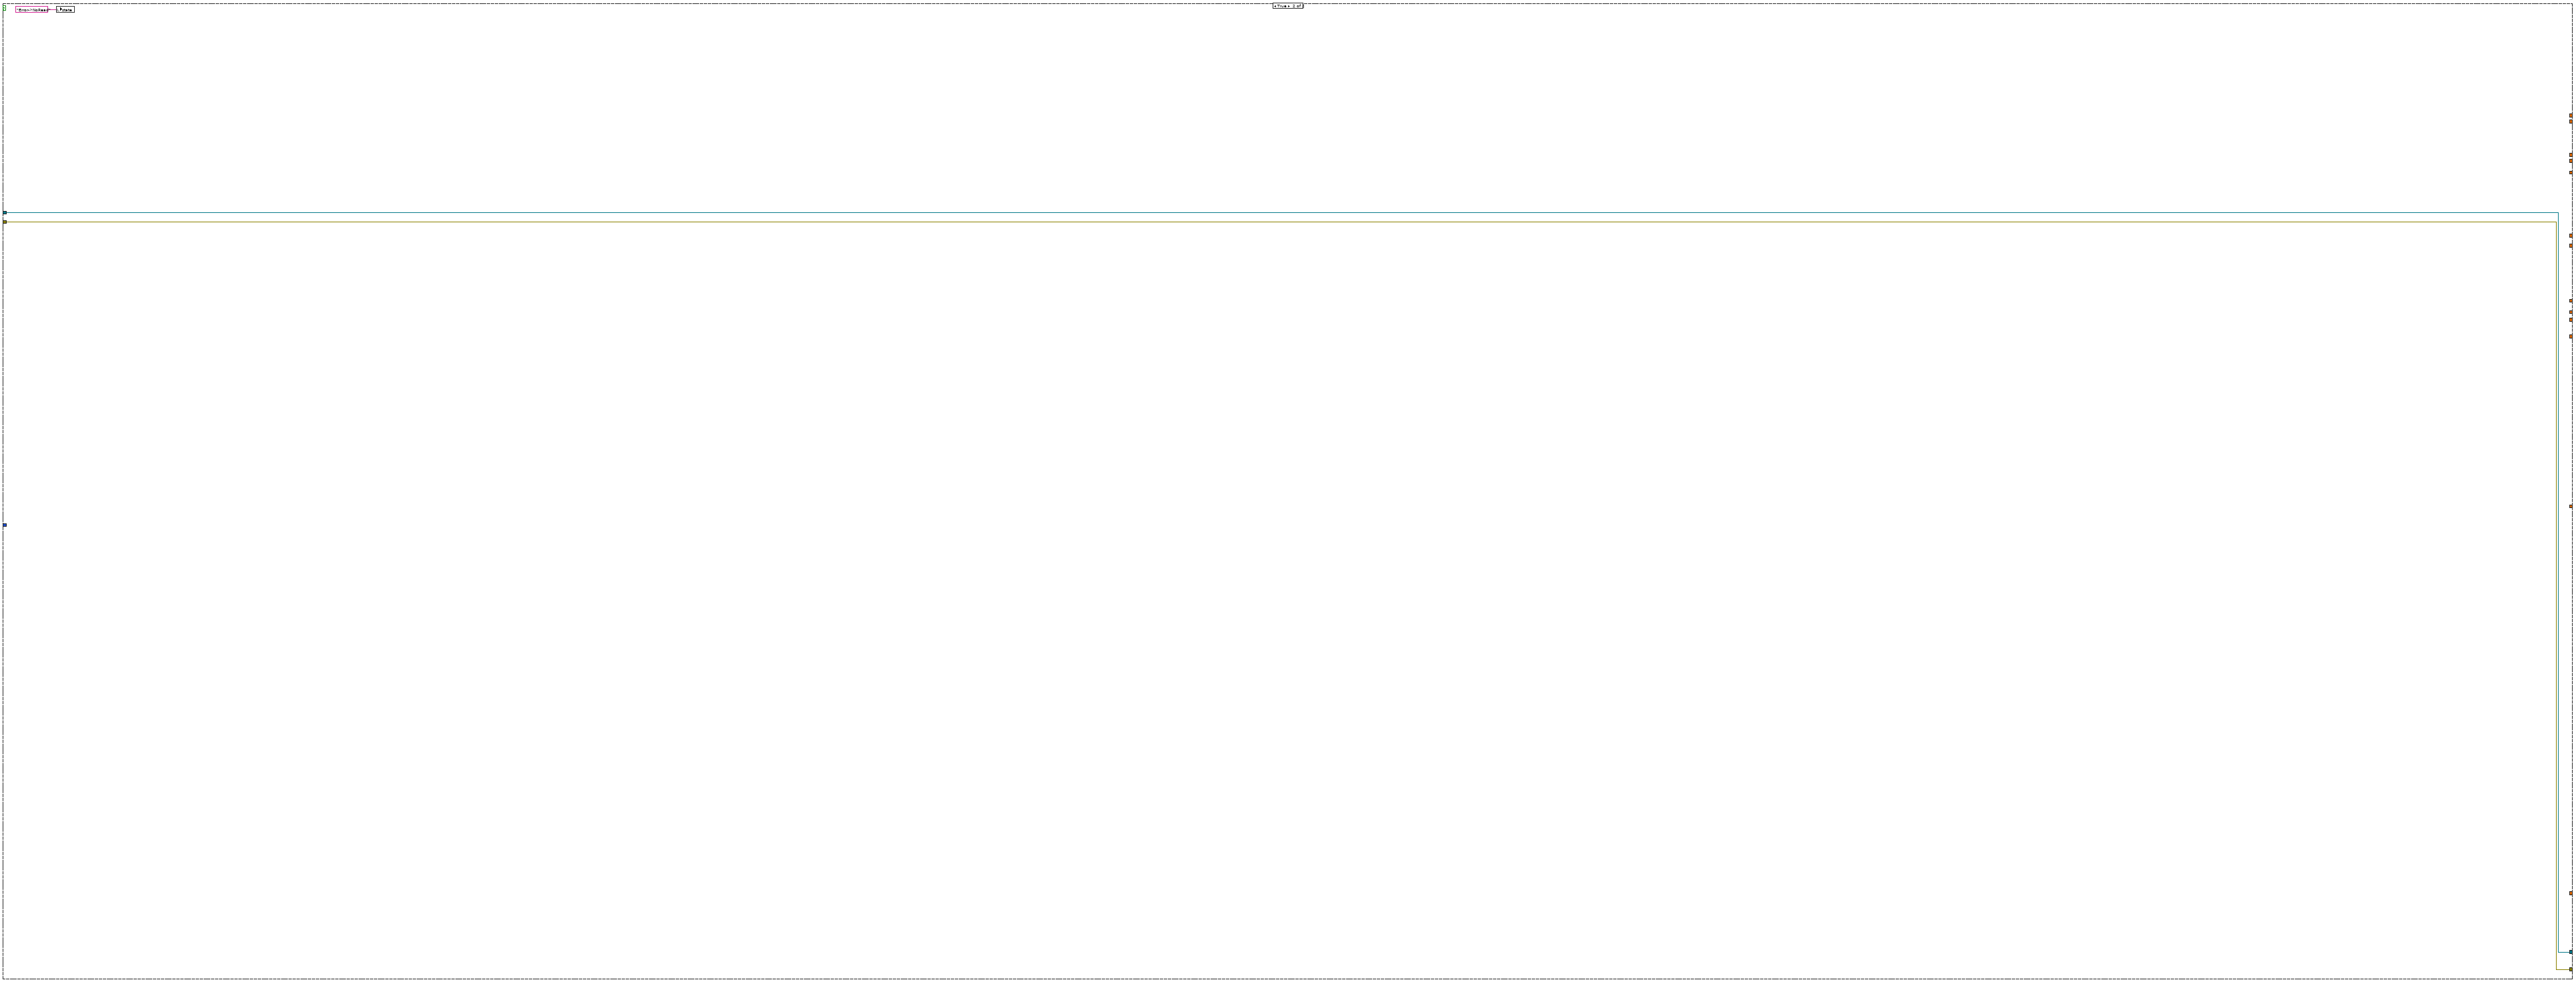
[diagram p12: hidden frame]
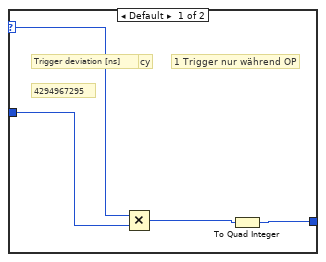
[diagram p13: hidden frame]
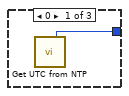
[diagram p14: hidden frame]
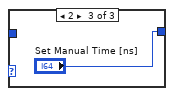
[diagram p15: hidden frame]
diagram:
  w11 = i64 -1  # Time Array needs to be positive!
  w30 = i64 -1000000000  # Ns per Sec
  w68 = 1 ("sampleCount")
  w69 = 1 ("sampleCount")
  w72 = "s"  # Unit
  w93 = "V"  # Unit
  w97 = "A"  # Unit
  w7 = "A"  # Unit
  w101 = "A"  # Unit
  w108 = 1 ("sampleCount")
  w110 = 1 ("sampleCount")
  w112 = 1 ("sampleCount")
  w67 = 1 ("sampleCount")
  w36 = 1 ("sampleCount")
  w118 = "Float"  # datatype
  w88 = "mV"  # Unit
  w90 = "Offset"  # label
  w124 = "Float"  # datatype
  w85 = "W"  # Unit
  w87 = "RKappa"  # label
  w126 = "Float"  # datatype
  w82 = "Ohms"  # Unit
  w84 = "RRes"  # label
  w128 = "Float"  # datatype
  w79 = "s"  # Unit
  w81 = "RTau"  # label
  w130 = "Float"  # datatype
  w76 = "W"  # Unit
  w78 = "MKappa"  # label
  w132 = "Float"  # datatype
  w75 = "Ohms"  # Unit
  w74 = "MRes"  # label
  w134 = "Float"  # datatype
  w71 = "MTau"  # label
  w37 = 10000 ("dimension size")
  w142 = 10000 ("sampleCount")
  w144 = "Float"  # datatype
  w103 = "A"  # Unit
  w105 = "BoloCalibRefFoilFit"  # label
  w145 = 10000 ("sampleCount")
  w147 = "Float"  # datatype
  w99 = "BoloCalibRefFoilCurrent"  # label
  w148 = 10000 ("sampleCount")
  w150 = "Float"  # datatype
  w6 = "BoloCalibMeasFoilFit"  # label
  w151 = 10000 ("sampleCount")
  w153 = "Float"  # datatype
  w95 = "BoloCalibMeasFoilCurrent"  # label
  w155 = "Float"  # datatype
  w92 = "BoloSignal"  # label
  # "Negative Sample Time [ns]"
  # "Time array for Bolo Signal"
  # "No of Samples DAQ"
  # "Time array for Bolo Signal"
  # "+ wait Time"
  # "-800000ns for 0.8ms"
  # "Negative Sample Time [ns]"
  # "Here Changed Names"
  # "Time Stamp for JSON Files"
  # "Sample rate for Calibration Arrays\n should be hardwired to calirbation settings"
  # "Sample Rate in [ns]"
  # "Calculated Start Time [ns]"
  # "NSample"
  # "10000"
  # "Initialize Array:\nDimesions Size = NSamples"
  # "Pulselength fixed for 0.4ms sample time and 10000 samples"
  # "NSamples * SampleTime = PulseLength"
  # "Data here is incorrect as well=!"
  # "Sample Time [s]\ncalculated to \nSample Time [ns]"
  # "Creating virtual Time Stamp\nfor Shot and for Calibration (Hardwired to 10000 samples)\nShot is depending on set sample rate"
  # "Index von dem Sample\nals der Trigger empfangen wurde"
  # "T1 Trigger\nkommt hier"
  # "A=> Internal full scale calibration\n8=> Internal zero scale calibration\nC=> System Zero scale Calibration\n2=> Continuous conversion\n\n5V reference\n80 mV scale\nChannel 1 input (voltage at bridge)\nMaster clock disable\n\np.15 7730 manual"
  # "AC 1.25 kHz Frequenz\nSKIP=0"
  n1 = flat-sequence {
    tunnel: [w214] -> w55
    tunnel: ["FPGA VI Reference In"] -> w60
    tunnel: [w215] -> w58
    tunnel: w55 -> [w215]
    frame #0 {
      n2 = Tick Count (ms)() -> (millisecond timer value=w214:u32)
    }
    frame #1 {
      n3 = case shown="True" "Clear all Values \nfrom Beginning" {
        frame False {
        }
        frame True {
          n4 = flat-sequence {
            frame #0 {
              w219 = bool[] [] ("MessStatus 1-32")
              w218 = dbl[] [] ("Kappa00")
              w221 = T20 {"tstart"=0.0, "dt"=0.0, "OutArray"=[]} ("Channels 9 - 12")
              # "Clear Graphs"
              n5 = local write "RREF"(w218) -> ()
              n6 = local write "Kappa00"(w218) -> ()
              n7 = local write "TauR"(w218) -> ()
              n8 = local write "Tau00"(w218) -> ()
              n9 = local write "RB000"(w218) -> ()
              n10 = local write "RefStatus 97-128"(w219) -> ()
              n11 = local write "RefStatus 1-32"(w219) -> ()
              n12 = local write "RefStatus 33-64"(w219) -> ()
              n13 = local write "RefStatus 65-96"(w219) -> ()
              n14 = local write "KappaR"(w218) -> ()
              n15 = local write "RMESS"(w218) -> ()
              n16 = local write "MessStatus 1-32"(w219) -> ()
              n17 = local write "MessStatus 33-64"(w219) -> ()
              n18 = local write "MessStatus 65-96"(w219) -> ()
              n19 = local write "MessStatus 97-128"(w219) -> ()
              n20 = local write "KappaM"(w218) -> ()
              n21 = local write "TauM"(w218) -> ()
              n22 = local write "DACbits 2"(w218) -> ()
              n23 = Bundle("Channels 9 - 12"=w221, "Channels 9 - 12"=w221, "Channels 9 - 12"=w221, "Channels 9 - 12"=w221) -> (w220:T21)  [unwired: 1 in]
              n24 = local write "Raw 1-32"(w220) -> ()
              n25 = local write "Raw 33-64"(w220) -> ()
              n26 = local write "Pow 1-32"(w220) -> ()
              n27 = local write "Pow 33-64"(w220) -> ()
              n28 = local write "RangeIndex"(w218) -> ()
              n29 = local write "Mean (mV)"(w218) -> ()
              n30 = local write "Peak to Peak \n      (microV)"(w218) -> ()
              n31 = local write "StandardDeviation\n        (microV)"(w218) -> ()
              n32 = local write "Raw 65 - 97"(w220) -> ()
              n33 = local write "Raw 97 - 128"(w220) -> ()
              n34 = local write "Offset 1-32"(w220) -> ()
              n35 = local write "Offset 33-64"(w220) -> ()
              n36 = local write "Offset 65 - 96"(w220) -> ()
              n37 = local write "Offset 97 - 128"(w220) -> ()
              n38 = local write "RefCal 1-16"(w220) -> ()
              n39 = local write "RefCal 113 - 128"(w220) -> ()
              n40 = local write "RefCal 17-32"(w220) -> ()
              n41 = local write "RefCal 33 - 48"(w220) -> ()
              n42 = local write "RefCal 49 - 64"(w220) -> ()
              n43 = local write "RefCal 65 - 80"(w220) -> ()
              n44 = local write "RefCal 81 - 96"(w220) -> ()
              n45 = local write "RefCal 97 - 112"(w220) -> ()
              n46 = local write "Pow 65 - 96"(w220) -> ()
              n47 = local write "Pow 97 - 128"(w220) -> ()
              n48 = local write "MessCal 1-16"(w220) -> ()
              n49 = local write "MessCal 113 - 128"(w220) -> ()
              n50 = local write "MessCal 17-32"(w220) -> ()
              n51 = local write "MessCal 33 - 49"(w220) -> ()
              n52 = local write "MessCal 49 - 64"(w220) -> ()
              n53 = local write "MessCal 65 - 80"(w220) -> ()
              n54 = local write "MessCal 81 - 96"(w220) -> ()
              n55 = local write "MessCal 97 - 112"(w220) -> ()
            }
          }
        }
      }
    }
  }
  n56 = Not A Number/Path/Refnum?(number/path/refnum=w60) -> (NaN/Path/Refnum?=w59:bool)
  n57 = case shown="True" w59 {
    tunnel: [w222 w224] -> w172
    tunnel: [_ w223] -> w171
    tunnel: w60 -> [w222 _]
    frame False {
    }
    frame True {
      n58 = xnode "Open FPGA VI Reference"("resource name"=T22 "RIO0") -> ("FPGA VI Reference Out"=w224:refnum<k20>, "error out"=w223:errorcluster)  [unwired: 1 in]
    }
  }
  "error out" <- w171
  n59 = flat-sequence {
    tunnel: "Cancel" ("name (unnamed)") -> [w235]
    tunnel: "Transferred1" ("name (unnamed)") -> [w234]
    tunnel: u32 0 -> [w233]
    tunnel: FALSE -> [w232]
    tunnel: [w231] -> w204
    tunnel: [w230] -> w203
    tunnel: [w229] -> w202
    tunnel: [w228] -> w201
    tunnel: [u32 0] -> w63
    frame #0 {
      n60 = local write "stop"(FALSE ("stop")) -> ()
      n61 = RT FIFO Create(0:w234, 1:w233) -> (8:w228:refnum<k33>, 11:w229:errorcluster)  [unwired: 2 in, 5 out]
      n62 = RT FIFO Create(0:w235, 1:w232) -> (8:w231:refnum<k33>, 11:w230:errorcluster)  [unwired: 3 in, 4 out]
    }
  }
  n63 = xnode "Read/Write Control"("FPGA VI Reference In"=w172, "error in"=w171, "cancel"=TRUE ("clrFifo"), "Test"=FALSE) -> ("FPGA VI Reference Out"=w213:refnum<k20>, "error out"=w212:errorcluster)
  n64 = flat-sequence {
    tunnel: w213 -> [w242]
    tunnel: w212 -> [w241]
    tunnel: [w240] -> w211
    tunnel: [w239] -> w210
    frame #0 {
      n65 = Wait (ms)(milliseconds to wait=u32 100) -> ()  [unwired: 1 out]
      n66 = xnode "Invoke Method"("FPGA VI Reference In"=w242, "error in"=w241, "IRQ Number(s)"=i32[] [0, 1, 2, 3]) -> ("FPGA VI Reference Out"=w240:refnum<k20>, "error out"=w239:errorcluster)
      "state" <- "Start (100 ms)" ("state")
    }
  }
  n67 = node-c288() -> (w196:T23)  [unwired: 1 in, 4 out]
  n68 = timed-loop {
    tunnel: w204 -> [w253]
    tunnel: w203 -> [w252]
    tunnel: w202 -> [w251]
    tunnel: w201 -> [w250]
    shift-right: [w249] -> _
    shift-left: w63 -> [w243]
    tunnel: [w248] -> w198
    tunnel: [w247] -> w197
    tunnel: [w246] -> w200
    tunnel: [w245] -> w199
    timing: w196 -> [_]
    timing-out: [_] -> w195
    stop <- "stop" stop-if-true
    n69 = RT FIFO Read(0:w250, 1:w243, 3:w251) -> (8:w246:refnum<k33>, 9:w249:u32, 11:w245:errorcluster)  [unwired: 3 out]
    n70 = RT FIFO Write(0:w253, 1:"Cancel Button", 3:w252) -> (8:w248:refnum<k33>, 11:w247:errorcluster)  [unwired: 1 in, 3 out]
    "Acquired Samples:" <- w243
  }
  n71 = flat-sequence {
    tunnel: w210 -> [w258]
    tunnel: [w257] -> w192
    tunnel: w211 -> [w259]
    tunnel: [w260] -> w174
    frame #0 {
      n72 = local write "state"("Reset" ("state")) -> ()
      n73 = call "hReset2014.vi"("error in"=w258, "FPGA VI Reference In"=w259) -> ("error out"=w257:errorcluster, "FPGA VI Reference Out"=w260:refnum<k20>)  [unwired: 4 in]
    }
  }
  n74 = node-c288(w195) -> ()  [unwired: 1 out]
  n75 = call "hFilterReg2014.vi"("error in"=w192, "Filter Modus"=u16 61 ("t"), "Frequenz"=u8 79 ("AC 1kHz Frequenz\nSKIP=0"), "FPGA VI Reference In"=w174) -> ("error out"=w177:errorcluster, "Timed Out"=w186:bool, "FPGA VI Reference Out"=w176:refnum<k20>)  [unwired: 1 in]
  "FilterTimeOut" <- w186
  n76 = flat-sequence {
    tunnel: w200 -> [w266]
    tunnel: w199 -> [w265]
    tunnel: w198 -> [w264]
    tunnel: w197 -> [w263]
    frame #0 {
      n77 = RT FIFO Delete(0:w266, 3:w265) -> ()  [unwired: 1 in, 1 out]
      n78 = RT FIFO Delete(0:w264, 3:w263) -> ()  [unwired: 1 in, 1 out]
      n79 = local write "stop"(FALSE ("stop")) -> ()
    }
  }
  n80 = call "hModeReg2014.vi"("error in"=w177, "Mode"=u16 41144, "FPGA VI Reference In"=w176) -> ("error out"=w180:errorcluster, "Timeout"=w190:bool, "FPGA VI Reference Out"=w183:refnum<k20>)  [unwired: 2 in]
  n81 = call "hModeReg2014.vi"("error in"=w180, "Mode"=u16 32952, "FPGA VI Reference In"=w183) -> ("error out"=w179:errorcluster, "Timeout"=w191:bool, "FPGA VI Reference Out"=w182:refnum<k20>)  [unwired: 2 in]
  n82 = call "hModeReg2014.vi"("error in"=w179, "Mode"=u16 8376, "FPGA VI Reference In"=w182) -> ("error out"=w188:errorcluster, "Timeout"=w189:bool, "FPGA VI Reference Out"=w187:refnum<k20>)  [unwired: 2 in]
  n83 = Compound Arithmetic op=OR(w190, w191, w189, w186) -> (w175:bool)
  "result" <- w175
  n84 = case shown="False" w175 {
    tunnel: [w284 w725] -> w56
    tunnel: [w282 w724] -> w209
    tunnel: w187 -> [w446 w725]
    tunnel: w188 -> [w445 w724]
    tunnel: [w304 _] -> w154
    tunnel: [w340 _] -> w140
    tunnel: [w335 _] -> w141
    tunnel: [w331 _] -> w138
    tunnel: [w328 _] -> w139
    tunnel: [w280 _] -> w61
    tunnel: [w326 _] -> w123
    tunnel: [w325 _] -> w62
    tunnel: [w324 _] -> w122
    tunnel: [w323 _] -> w121
    tunnel: [w302 _] -> w120
    tunnel: [w306 _] -> w12
    tunnel: w58 -> [w273 _]
    tunnel: [w267 _] -> w31
    frame False {
      w347 = 2000
      w360 = u8 125  # Frequenz
      w405 = 0.0008 ("FPGSampleTime")
      w400 = 0.0
      w272 = 40.0  # Rcable
      w440 = 10.0  # Rload
      w460 = sgl 0.0004  # dt
      w461 = sgl 0.0  # tstart
      w464 = sgl 0.0004  # dt
      w465 = sgl 0.0  # tstart
      w469 = sgl 80.0 ("Scale(mV)")
      # "Offset Shift manually disabled because not need for low power discharges"
      # "Local TDMS Data Storage"
      # "Absolute Timer [ms] (Now)\n-\nAbsolute Timer [ms] (At Start)\n=\nTime need until start of DAQ"
      # "Startzeit - 14 s"
      # "old time from OP1"
      # "Store raw data"
      # "#Timing \n\nAC measurements\n2.083 kHz\nwith SKIP=1 \n\n= 5MHz/16/(3*45+15)"
      # "#Offset measurement"
      # "#Offset applied"
      # "#Range for measurements"
      # "A=> Internal full scale calibration\n8=> Internal zero scale calibration\nC=> System Zero scale Calibration\n2=> Continuous conversion\n\n2.5V reference\n80 mV scale\nChannel 2 input (voltage at shunt)\nMaster clock disable\n\np.15 7730 manual"
      n85 = flat-sequence {
        tunnel: [w559] -> w278
        tunnel: [w558] -> w277
        tunnel: w446 -> [w562]
        tunnel: w445 -> [w561]
        tunnel: w347 -> [w567]
        tunnel: [w566] -> w349
        tunnel: w278 -> [w569]
        tunnel: w277 -> [w568]
        tunnel: [w565] -> w348
        tunnel: [w575] -> w526
        tunnel: [w574] -> w525
        tunnel: [w573] -> w523
        tunnel: w347 -> [w571]
        tunnel: w349 -> [w577]
        tunnel: w348 -> [w576]
        frame #0 {
          n86 = call "hComRegStart2013.vi"("error in"=w561, "FPGA VI Reference In"=w562) -> ("error out"=w558:errorcluster, "Timed Out"=→"Timed Out 2":bool, "FPGA VI Reference Out"=w559:refnum<k20>)  [unwired: 3 in]
          n87 = call "Wait3"("Count(mSec)"=u32 3000) -> ()  [unwired: 1 out]
        }
        frame #1 {
          n88 = call "Wait6"("Count(mSec)"=u32 1000) -> ()  [unwired: 1 out]
          n89 = local write "state"("SyncRun (1000 ms)" ("state")) -> ()
          n90 = call "hSync&StartSampling2013.vi"("error in"=w568, "#Samples"=w567, "FPGA VI Reference In"=w569) -> ("error out"=w566:errorcluster, "FPGA VI Reference Out"=w565:refnum<k20>)  [unwired: 1 in]
        }
        frame #2 {
          n91 = call "hReadChannelsRTDMA2013.vi"("FPGA VI Reference In"=w576, "Nsamples"=w571, "error in"=w577) -> ("FPGA VI Reference Out"=w575:refnum<k20>, "Fehler"=→"Fehler":bool, "RawArray"=w573:i16[][], "error out"=w574:errorcluster)  [unwired: 2 in]
          n92 = local write "state"("ReadOffset" ("state")) -> ()
        }
      }
      n93 = property on="Acquired Samples:" class="Slide (strict)"("Scale.Range:Maximum"=w347) -> ()  [unwired: 2 in, 2 out]
      n94 = call "hSoftReset2013.vi"("error in"=w525, "FPGA VI Reference In"=w526) -> ("error out"=w358:errorcluster, "FPGA VI Reference Out"=w351:refnum<k20>)  [unwired: 4 in]
      n95 = call "Int2Volt2D.vi"("IntegerArray"=w523, "Scale(mV)"=sgl 80.0) -> ("RealArray"=w396:sgl[][])
      n96 = xnode "Read/Write Control"("FPGA VI Reference In"=w351, "error in"=w358, "HIREF"=TRUE) -> ("FPGA VI Reference Out"=w354:refnum<k20>, "error out"=w353:errorcluster)
      n97 = for {
        tunnel: w396 -> [w598] mode=indexing
        tunnel: [w597] -> w393 mode=indexing
        tunnel: [w596] -> w395 mode=indexing
        tunnel: [w595] -> w394 mode=indexing
        n98 = Array Subset(array=w598, index=500, length=1000) -> (w600:sgl[])
        n99 = Array Max & Min(array=w600) -> (max value=w603:sgl, min value=w604:sgl)  [unwired: 2 out]
        n100 = Subtract(x=w603, y=w604) -> (x-y=w597:sgl)
        n101 = call <vilib>:"Std Deviation and Variance.vi"("X"=w600, "Weighting (Sample)"=enum16{"Sample", "Population"}."Population") -> ("mean"=w596:dbl, "standard deviation"=w595:dbl)  [unwired: 1 out]
      }
      n102 = Array Subset(array=w396, index (row)=0, length (row)=64, index (col)=0) -> (w410:sgl[][])  [unwired: 1 in]
      n103 = Array Subset(array=w396, index (row)=64, length (row)=64, index (col)=0) -> (w406:sgl[][])  [unwired: 1 in]
      n104 = call "Visualize_Signals64.vi"("FPGSampleTime"=w405, "tstart"=w400, "Signals"=w410) -> ("plot(Signals) 33-64"=→"Offset 33-64":T26, "plot(Signals) 1-32"=→"Offset 1-32":T5)  [unwired: 7 in]
      n105 = call "Visualize_Signals64.vi"("FPGSampleTime"=w405, "tstart"=w400, "Signals"=w406) -> ("plot(Signals) 33-64"=→"Offset 97 - 128":T26, "plot(Signals) 1-32"=→"Offset 65 - 96":T5)  [unwired: 7 in]
      n106 = call "hFilterReg2014.vi"("error in"=w353, "Filter Modus"=u16 512 ("t"), "Frequenz"=w360, "FPGA VI Reference In"=w354) -> ("error out"=w352:errorcluster, "FPGA VI Reference Out"=w355:refnum<k20>)  [unwired: 1 in, 1 out]
      n107 = call "hModeReg2014.vi"("error in"=w352, "Mode"=u16 41017, "FPGA VI Reference In"=w355) -> ("error out"=w364:errorcluster, "FPGA VI Reference Out"=w363:refnum<k20>)  [unwired: 2 in, 1 out]
      n108 = call "hModeReg2014.vi"("error in"=w364, "Mode"=u16 32825, "FPGA VI Reference In"=w363) -> ("error out"=w361:errorcluster, "FPGA VI Reference Out"=w362:refnum<k20>)  [unwired: 2 in, 1 out]
      n109 = call "hModeReg2014.vi"("error in"=w361, "Mode"=u16 8249, "FPGA VI Reference In"=w362) -> ("error out"=w356:errorcluster, "FPGA VI Reference Out"=w357:refnum<k20>)  [unwired: 2 in, 1 out]
      n110 = Multiply(x=w394, y=1000000.0 ("Scale")) -> (x*y=→"StandardDeviation\n        (microV)":dbl[])
      n111 = Multiply(x=w393, y=1000000.0 ("Scale")) -> (x*y=→"Peak to Peak \n      (microV)":dbl[])
      n112 = Multiply(x=w395, y=1000.0 ("Scale")) -> (x*y=w306:dbl[])
      "Mean (mV)" <- w306
      n113 = control-ref of="Acquired Samples:"() -> (w520:refnum<vi>)
      n114 = control-ref of="Cancel Button"() -> (w522:refnum<vi>)
      n115 = control-ref of="state"() -> (w521:refnum<vi>)
      n116 = call "hCalRT2013.vi"("FPGA VI Reference In"=w357, "cancelbutton"=w522, "state"=w521, "Acquired Samples"=w520, "error in"=w356) -> ("FPGA VI Reference Out"=w443:refnum<k20>, "Ref"=w468:i16[][], "Meas"=w518:i16[][], "error out"=w442:errorcluster)  [unwired: 6 in, 1 out]
      "error out Cal" <- w442
      n117 = call "Int2Volt2D.vi"("IntegerArray"=w468, "Scale(mV)"=w469) -> ("RealArray"=w470:sgl[][])
      n118 = call "Int2Volt2D.vi"("IntegerArray"=w518, "Scale(mV)"=w469) -> ("RealArray"=w519:sgl[][])
      n119 = flat-sequence {
        tunnel: w443 -> [w588]
        tunnel: w442 -> [w586]
        tunnel: [w587] -> w369
        tunnel: [w585] -> w368
        tunnel: [w592] -> w321
        tunnel: [w591] -> w399
        tunnel: w369 -> [w594]
        tunnel: w368 -> [w593]
        frame #0 {
          w582 = FALSE ("RESET")
          n120 = call "Wait"("Count(mSec)"=u16 3000 ("Count(uSec)")) -> ()  [unwired: 1 out]
          n121 = xnode "Read/Write Control"("FPGA VI Reference In"=w588, "error in"=w586, "RLY1"=w582, "RLY2"=w582, "HIREF"=w582, "Sprung0"=w582, "Sprung1"=w582, "ScanID"=u32 0, "Test"="Switch to fixed \nCalibration Values", "RESET"=TRUE) -> ("FPGA VI Reference Out"=w587:refnum<k20>, "error out"=w585:errorcluster)
          n122 = local write "state"("SoftReset (3000 ms)" ("state")) -> ()
        }
        frame #1 {
          n123 = xnode "Read/Write Control"("FPGA VI Reference In"=w594, "error in"=w593, "RESET"=FALSE) -> ("FPGA VI Reference Out"=w591:refnum<k20>, "error out"=w592:errorcluster)
          n124 = call "Wait5"("Count(mSec)"=u16 1000 ("Count(uSec)")) -> ()  [unwired: 1 out]
        }
      }
      n125 = case shown="True" "SecondFilter" {
        tunnel: [w539 w548] -> w267
        tunnel: [w538 w546] -> w346
        tunnel: [w537 w547] -> w345
        frame False {
          # "#Timing \n\nAC measurements\n2.5 kHz\nwith SKIP=1 \n\n= 5MHz/16/(3*37+14)"
          n126 = disable-structure shown="Enabled" {
            disable-tunnel: [u16 574 ("t") u16 575 ("t")] -> w537
            disable-tunnel: [u16 37 ("frequenz") u16 45 ("frequenz")] -> w538
            disable-tunnel: [sgl 0.0004 sgl 0.00048] -> w539
            frame Enabled {
            }
            frame Disabled {
            }
          }
        }
        frame True {
          # "#Timing \n\nAC measurements\n1.25 kHz\nwith SKIP=0 \n\n= 5MHz/16/250"
          n127 = call "FreqSel.vi"("Ring"="FreqSelRing") -> ("Frequency"=w546:u16, "DLY"=w547:u16, "SampleTime"=w548:sgl)  [unwired: 1 out]
        }
      }
      "SampleTime" <- w267
      n128 = xnode "Invoke Method"("FPGA VI Reference In"=w399, "error in"=w321, "Requested Depth"=u32 256) -> ("FPGA VI Reference Out"=w322:refnum<k20>, "error out"=w320:errorcluster, "Actual Depth"=→"Actual Depth":u32)
      n129 = call-poly <vilib>:"Read From Spreadsheet File.vi"("file path (dialog if empty)"="file path (dialog if empty)") -> ("first row"=w269:i64[])  [unwired: 6 in, 4 out]
      n130 = call "hFilterReg2014.vi"("error in"=w320, "Filter Modus"=w345, "Frequenz"=w346, "FPGA VI Reference In"=w322) -> ("error out"=w459:errorcluster, "FPGA VI Reference Out"=w458:refnum<k20>)  [unwired: 1 in, 1 out]
      n131 = To Unsigned Byte Integer(number=w269) -> (unsigned 8bit integer=w268:u8[])
      "RangeIndex" <- w268
      n132 = case shown="True" "Global or Individual\nDAC Settings loaded \nfrom File" {
        tunnel: w459 -> [w693 w709]
        tunnel: w458 -> [w694 w708]
        tunnel: [w688 w707] -> w397
        tunnel: [w691 w699] -> w398
        tunnel: u16 41096 -> [w686 w698]
        tunnel: u16 49288 -> [_ w700]
        tunnel: u16 8328 -> [w687 w696]
        tunnel: w268 -> [w685 _]
        tunnel: u16 32904 -> [w683 w697]
        frame False {
          # "MIddle Previously connected xC088 not to x8088"
          n133 = call "hModeRegRange2013.vi"("error in"=w693, "RangeArray"=w685, "Mode"=w686, "FPGA VI Reference In"=w694) -> ("error out"=w690:errorcluster, "FPGA VI Reference Out"=w692:refnum<k20>)  [unwired: 1 in, 1 out]
          n134 = call "hModeRegRange2013.vi"("error in"=w690, "RangeArray"=w685, "Mode"=w683, "FPGA VI Reference In"=w692) -> ("error out"=w689:errorcluster, "FPGA VI Reference Out"=w684:refnum<k20>)  [unwired: 1 in, 1 out]
          n135 = call "hModeRegRange2013.vi"("error in"=w689, "RangeArray"=w685, "Mode"=w687, "FPGA VI Reference In"=w684) -> ("error out"=w688:errorcluster, "FPGA VI Reference Out"=w691:refnum<k20>)  [unwired: 1 in, 1 out]
        }
        frame True {
          n136 = call "hModeReg2014.vi"("error in"=w709, "Range"="DAC Range Setting", "Mode"=w698, "FPGA VI Reference In"=w708) -> ("error out"=w705:errorcluster, "FPGA VI Reference Out"=w706:refnum<k20>)  [unwired: 1 in, 1 out]
          n137 = call "hModeReg2014.vi"("error in"=w705, "Range"="DAC Range Setting", "Mode"=w697, "FPGA VI Reference In"=w706) -> ("error out"=w703:errorcluster, "FPGA VI Reference Out"=w704:refnum<k20>)  [unwired: 1 in, 1 out]
          n138 = disable-structure shown="Enabled" {
            disable-tunnel: w704 -> [w715 w717]
            disable-tunnel: w703 -> [w714 w716]
            disable-tunnel: [w713 w717] -> w702
            disable-tunnel: [w712 w716] -> w701
            disable-tunnel: w700 -> [w711 _]
            disable-tunnel: "DAC Range Setting" -> [w710 _]
            frame Disabled {
              n139 = call "hModeReg2014.vi"("error in"=w714, "Range"=w710, "Mode"=w711, "FPGA VI Reference In"=w715) -> ("error out"=w712:errorcluster, "FPGA VI Reference Out"=w713:refnum<k20>)  [unwired: 1 in, 1 out]
            }
            frame Enabled {
            }
          }
          n140 = call "hModeReg2014.vi"("error in"=w701, "Range"="DAC Range Setting", "Mode"=w696, "FPGA VI Reference In"=w702) -> ("error out"=w707:errorcluster, "FPGA VI Reference Out"=w699:refnum<k20>)  [unwired: 1 in, 1 out]
        }
      }
      n141 = disable-structure shown="Enabled" {
        disable-tunnel: w398 -> [w555 w556]
        disable-tunnel: w397 -> [w554 w557]
        disable-tunnel: w268 -> [w553 _]
        disable-tunnel: [w552 _] -> w376
        disable-tunnel: [w551 w556] -> w371
        disable-tunnel: [w550 w557] -> w315
        frame Disabled {
          n142 = call "hDACsubtract2013.vi"("FPGA VI Reference In"=w555, "Ranges"=w553, "error in"=w554) -> ("FPGA VI Reference Out"=w551:refnum<k20>, "DACbits"=w552:u16[], "error out"=w550:errorcluster)  [unwired: 10 in]
        }
        frame Enabled {
        }
      }
      n143 = property on="Acquired Samples:" class="Slide (strict)"(error in=w315, "Scale.Range:Maximum"="No. of Samples:") -> (error out=w314:errorcluster)  [unwired: 1 in, 1 out]
      n144 = Subtract(x=w376, y=u16 1024 ("NSample")) -> (x-y=→"DACbits 2":u16[])
      n145 = flat-sequence {
        tunnel: w314 -> [w607]
        tunnel: w371 -> [w609]
        tunnel: [w608] -> w317
        tunnel: [w606] -> w316
        tunnel: w317 -> [w623]
        tunnel: [w623] -> w311
        tunnel: w316 -> [w622]
        tunnel: [w622] -> w309
        tunnel: w273 -> [w611]
        tunnel: w311 -> [w632]
        tunnel: [w631] -> w310
        tunnel: w309 -> [w630]
        tunnel: [w629] -> w308
        tunnel: "No. of Samples:" -> [w628]
        tunnel: w310 -> [w633]
        tunnel: w308 -> [w634]
        tunnel: w273 -> [w635]
        tunnel: [w633] -> w299
        tunnel: [w634] -> w298
        tunnel: w299 -> [w641]
        tunnel: w298 -> [w640]
        tunnel: [w641] -> w297
        tunnel: [w640] -> w296
        tunnel: [w639] -> w295
        tunnel: w297 -> [w653]
        tunnel: w296 -> [w654]
        tunnel: w295 -> [w647]
        tunnel: "No. of Samples:" -> [w652]
        tunnel: w294 -> [w651]
        tunnel: w293 -> [w650]
        tunnel: w292 -> [w649]
        tunnel: w271 -> [w648]
        tunnel: [w646] -> w291
        tunnel: [w647] -> w290
        tunnel: [w645] -> w289
        tunnel: [w644] -> w288
        tunnel: [w643] -> w287
        tunnel: [w642] -> w286
        tunnel: [w678] -> w282
        tunnel: [w679] -> w344
        tunnel: [w680] -> w283
        tunnel: [w681] -> w284
        tunnel: [w682] -> w373
        tunnel: w290 -> [w682]
        tunnel: w289 -> [w681]
        tunnel: w288 -> [w680]
        tunnel: w287 -> [w679]
        tunnel: w286 -> [w678]
        tunnel: [w676] -> w285
        frame #0 {
          n146 = call "hComRegStart2013.vi"("error in"=w607, "FPGA VI Reference In"=w609) -> ("error out"=w606:errorcluster, "FPGA VI Reference Out"=w608:refnum<k20>)  [unwired: 3 in, 1 out]
          n147 = local write "state"("Calibration Done" ("state")) -> ()
          n148 = call "Wait4"("Count(mSec)"=u32 1000) -> ()  [unwired: 1 out]
        }
        frame #1 {
          (unwired) 15000  # fixed -15sec for T0
          w614 = 60000  # fixed -60sec before T1 = T0
          n149 = Subtract(x=w614, y="Pre-start time (ms) of DAQ \nTypically set to 1000 ms") -> (x-y=w615:i32)
          "Total wait time (TWT)\nTypically 59 s" <- w615
          n150 = Add(x=w611, y=w615) -> (x+y=w612:u32)
          n151 = Tick Count (ms)() -> (millisecond timer value=w617:u32)
          n152 = Subtract(x=w612, y=w617) -> (x-y=w618:u32)
          "Calibration Time" <- w618
          n153 = Subtract(x=w618, y=u32 50) -> (x-y=w619:u32)
          "Countdown Time" <- w619
          n154 = Add(x=w617, y=w619) -> (x+y=w620:u32)
          n155 = while {
            tunnel: w620 -> [w626]
            stop <- w627 continue-if-true
            n156 = Tick Count (ms)() -> (millisecond timer value=w625:u32)
            n157 = Subtract(x=w626, y=w625) -> (x-y=w624:u32)
            "DAQ Timer" <- w624
            n158 = Greater?(x=w626, y=w625) -> (0:w627:bool)
            n159 = local write "DAQ Timer"(w624) -> ()
          }
          n160 = local write "state"("Countdown Timer" ("state")) -> ()
          "Fixed T-60sec before T1 = T0" <- w614
        }
        frame #2 {
          # "takes 50 ms"
          n161 = call "hSync&StartSampling2013.vi"("error in"=w630, "#Samples"=w628, "FPGA VI Reference In"=w632) -> ("error out"=w629:errorcluster, "FPGA VI Reference Out"=w631:refnum<k20>)  [unwired: 1 in]
        }
        frame #3 {
          n162 = Tick Count (ms)() -> (millisecond timer value=w636:u32)
          n163 = local write "state"("SyncRun" ("state")) -> ()
          n164 = Subtract(x=w636, y=w635) -> (x-y=→"DAQ wait time (should be = TWT":u32)
        }
        frame #4 {
          n165 = call "Tick Count"() -> ("Tick Count(mSec)"=w639:u32)
        }
        frame #5 {
          n166 = disable-structure shown="Enabled" {
            disable-tunnel: w654 -> [w667 w674]
            disable-tunnel: w653 -> [w666 w675]
            disable-tunnel: w652 -> [w665 w673]
            disable-tunnel: [w664 w672] -> w645
            disable-tunnel: [w663 w671] -> w642
            disable-tunnel: [w662 _] -> w646
            disable-tunnel: w649 -> [w661 _]
            disable-tunnel: w650 -> [w660 _]
            disable-tunnel: [w659 _] -> w644
            disable-tunnel: [w658 w669] -> w643
            disable-tunnel: w651 -> [w657 _]
            disable-tunnel: w648 -> [w656 _]
            frame Enabled {
              n167 = call "hReadChannels-UandP-2013.vi"("RawScal"=w660, "SumScal"=w661, "Scale(mV)"=w656, "Tau/dt"=w657, "error in"=w667, "Nsamples"=w665, "FPGA VI Reference In"=w666) -> ("error out"=w663:errorcluster, "RawArray"=w658:sgl[][], "PowerArray"=w659:sgl[][], "FPGA VI Reference Out"=w664:refnum<k20>, "Fehler"=w662:bool)
            }
            frame Disabled {
              n168 = call "hReadChannelsRTDMA2013.vi"("FPGA VI Reference In"=w675, "Nsamples"=w673, "error in"=w674) -> ("FPGA VI Reference Out"=w672:refnum<k20>, "RawArray"=w670:i16[][], "error out"=w671:errorcluster)  [unwired: 2 in, 1 out]
              n169 = call "Int2Volt2D.vi"("IntegerArray"=w670, "Scale(mV)"=sgl 80.0) -> ("RealArray"=w669:sgl[][])
            }
          }
          n170 = local write "state"("Acquiring Data..." ("state")) -> ()
        }
        frame #6 {
          n171 = local write "state"("Acquiring done" ("state")) -> ()
          n172 = call "Tick Count2"() -> ("Tick Count(mSec)"=w676:u32)
        }
      }
      n173 = Divide(x=w519, y=w440) -> (x/y=w332:dbl[][])
      n174 = call "CalFaktor-128.vi"("CalCurrent(t)"=w332, "Rload"=w440, "Rcable"=w272) -> ("FitData"=w327:dbl[][], "Kappa"=w280:dbl[], "Tau"=w325:dbl[], "RB01"=w326:dbl[])  [unwired: 1 out]
      "KappaM" <- w280
      n175 = Array Subset(array=w332, index (row)=0 ("index"), length (row)=128 ("length")) -> (w331:dbl[][])  [unwired: 2 in]
      n176 = Add(x=w272, y=w440) -> (x+y=w439:dbl)
      n177 = local read "Switch to fixed \nCalibration Values"() -> (w457:bool)
      n178 = Multiply(x=w439, y=2.0) -> (x*y=w437:dbl)
      n179 = case shown="False" w457 {
        tunnel: [w719 "RB000"] -> w441
        tunnel: [w718 "Kappa00"] -> w436
        tunnel: [w720 "Tau00"] -> w294
        tunnel: w325 -> [w720 _]
        tunnel: w326 -> [w719 _]
        tunnel: w280 -> [w718 _]
        frame False {
        }
        frame True {
        }
      }
      n180 = call "Cal(SubVI)-2013.vi"("Array"=w332, "dt"=w464, "StartChan"=64 ("ChanStart"), "tstart"=w465, "FitData"=w327) -> ("plot(Signals) 1-32"=→"MessCal 65 - 80":T27, "plot(Signals) 33-64"=→"MessCal 81 - 96":T28)  [unwired: 9 in]
      n181 = call "Cal(SubVI)-2013.vi"("Array"=w332, "dt"=w464, "StartChan"=96 ("ChanStart"), "tstart"=w465, "FitData"=w327) -> ("plot(Signals) 1-32"=→"MessCal 97 - 112":T27, "plot(Signals) 33-64"=→"MessCal 113 - 128":T28)  [unwired: 9 in]
      n182 = call "Cal(SubVI)-2013.vi"("Array"=w332, "dt"=w464, "StartChan"=32 ("ChanStart"), "tstart"=w465, "FitData"=w327) -> ("plot(Signals) 1-32"=→"MessCal 33 - 49":T27, "plot(Signals) 33-64"=→"MessCal 49 - 64":T28)  [unwired: 9 in]
      n183 = call "Cal(SubVI)-2013.vi"("Array"=w332, "dt"=w464, "StartChan"=0 ("ChanStart"), "tstart"=w465, "FitData"=w327) -> ("plot(Signals) 1-32"=→"MessCal 1-16":T27, "plot(Signals) 33-64"=→"MessCal 17-32":T28)  [unwired: 9 in]
      n184 = call "Arraylimit128.vi"("LowerLimit"=400.0, "Array Input"=w326, "UpperLimit"=2000.0) -> ("BoolArray"=w510:bool[], "ArrayOutput"=w279:dbl[])
      "RMESS" <- w279
      n185 = call "Arraylimit128.vi"("LowerLimit"=2e-05, "Array Input"=w280, "UpperLimit"=0.002) -> ("BoolArray"=w512:bool[])  [unwired: 1 out]
      n186 = call "Arraylimit128.vi"("LowerLimit"=0.001, "Array Input"=w325, "UpperLimit"=0.8) -> ("BoolArray"=w511:bool[], "ArrayOutput"=w281:dbl[])
      "TauM" <- w281
      n187 = call "U2PCoeff.vi"("Numeric"=w437, "Kappa00"=w436, "RB000"=w441) -> ("Array"=w293:dbl[], "Array 2"=w292:dbl[])
      n188 = Scale By Power Of 2(n=w268, x=sgl 10.0 ("Scale(mV)")) -> (x*2^n=w271:sgl[])
      n189 = Compound Arithmetic op=OR(w512, w511, w510) -> (w495:bool[])
      n190 = local read "Pre-start time (ms) of DAQ \nTypically set to 1000 ms"() -> (w313:i32)
      n191 = Array Subset(array=w495, index=0, length=32) -> (→"MessStatus 1-32":bool[])
      n192 = Array Subset(array=w495, index=32, length=32) -> (→"MessStatus 33-64":bool[])
      n193 = Array Subset(array=w495, index=64, length=32) -> (→"MessStatus 65-96":bool[])
      n194 = Array Subset(array=w495, index=96, length=32) -> (→"MessStatus 97-128":bool[])
      n195 = Divide(x=w470, y=w440) -> (x/y=w341:dbl[][])
      n196 = Divide(x=w313, y=sgl -1000.0 ("Scale(mV)")) -> (x/y=w276:sgl)
      "T-Start [for Display)\nShould be -1 [s]" <- w276
      n197 = call "CalFaktor-128.vi"("CalCurrent(t)"=w341, "Rload"=w440, "Rcable"=w272) -> ("FitData"=w274:dbl[][], "Kappa"=w302:dbl[], "Tau"=w323:dbl[], "RB01"=w324:dbl[])  [unwired: 1 out]
      "KappaR" <- w302
      n198 = Array Subset(array=w341, index (row)=0 ("index"), length (row)=128 ("length")) -> (w340:dbl[][])  [unwired: 2 in]
      n199 = call "Cal(SubVI)-2013.vi"("Array"=w341, "dt"=w460, "StartChan"=0 ("ChanStart"), "tstart"=w461, "FitData"=w274) -> ("plot(Signals) 1-32"=→"RefCal 1-16":T27, "plot(Signals) 33-64"=→"RefCal 17-32":T28)  [unwired: 9 in]
      n200 = call "Cal(SubVI)-2013.vi"("Array"=w341, "dt"=w460, "StartChan"=32 ("ChanStart"), "tstart"=w461, "FitData"=w274) -> ("plot(Signals) 1-32"=→"RefCal 33 - 48":T27, "plot(Signals) 33-64"=→"RefCal 49 - 64":T28)  [unwired: 9 in]
      n201 = call "Cal(SubVI)-2013.vi"("Array"=w341, "dt"=w460, "StartChan"=64 ("ChanStart"), "tstart"=w461, "FitData"=w274) -> ("plot(Signals) 1-32"=→"RefCal 65 - 80":T27, "plot(Signals) 33-64"=→"RefCal 81 - 96":T28)  [unwired: 9 in]
      n202 = call "Cal(SubVI)-2013.vi"("Array"=w341, "dt"=w460, "StartChan"=96 ("ChanStart"), "tstart"=w461, "FitData"=w274) -> ("plot(Signals) 1-32"=→"RefCal 97 - 112":T27, "plot(Signals) 33-64"=→"RefCal 113 - 128":T28)  [unwired: 9 in]
      n203 = Array Subset(array=w274, index (row)=0 ("index"), length (row)=128 ("length")) -> (w335:dbl[][])  [unwired: 2 in]
      n204 = call "Arraylimit128.vi"("LowerLimit"=400.0, "Array Input"=w324, "UpperLimit"=2000.0) -> ("BoolArray"=w479:bool[], "ArrayOutput"=w301:dbl[])
      "RREF" <- w301
      n205 = call "Arraylimit128.vi"("LowerLimit"=2e-05, "Array Input"=w302, "UpperLimit"=0.002) -> ("BoolArray"=w477:bool[])  [unwired: 1 out]
      n206 = call "Arraylimit128.vi"("LowerLimit"=0.001, "Array Input"=w323, "UpperLimit"=0.8) -> ("BoolArray"=w478:bool[], "ArrayOutput"=w303:dbl[])
      "TauR" <- w303
      n207 = Subtract(x=w285, y=w373) -> (x-y=→"Measured Time \nfor DAQ [ms] \nShould ~ correspond to\nSampleTime * Samples":u32)
      n208 = Compound Arithmetic op=OR(w477, w478, w479) -> (w494:bool[])
      n209 = Array Subset(array=w283, index (row)=64, length (row)=64, index (col)=0) -> (w426:sgl[][])  [unwired: 1 in]
      n210 = Array Subset(array=w283, index (row)=0, length (row)=64, index (col)=0) -> (w430:sgl[][])  [unwired: 1 in]
      n211 = Array Subset(array=w344, index (row)=64, length (row)=64, index (col)=0) -> (w305:sgl[][])  [unwired: 1 in]
      n212 = Array Subset(array=w344, index (row)=0, length (row)=64, index (col)=0) -> (w300:sgl[][])  [unwired: 1 in]
      n213 = Array Subset(array=w344, index (row)=0 ("index"), length (row)=128 ("length")) -> (w304:sgl[][])  [unwired: 2 in]
      n214 = Array Subset(array=w494, index=0, length=32) -> (→"RefStatus 1-32":bool[])
      n215 = Array Subset(array=w494, index=32, length=32) -> (→"RefStatus 33-64":bool[])
      n216 = Array Subset(array=w494, index=64, length=32) -> (→"RefStatus 65-96":bool[])
      n217 = Array Subset(array=w494, index=96, length=32) -> (→"RefStatus 97-128":bool[])
      n218 = disable-structure shown="Disabled" {
        disable-tunnel: w344 -> [w536 _]
        disable-tunnel: w303 -> [w535 _]
        disable-tunnel: w302 -> [w534 _]
        disable-tunnel: w301 -> [w533 _]
        disable-tunnel: w300 -> [w532 _]
        disable-tunnel: w281 -> [w531 _]
        disable-tunnel: w280 -> [w530 _]
        disable-tunnel: w279 -> [w529 _]
        disable-tunnel: w276 -> [w528 _]
        disable-tunnel: w267 -> [w527 _]
        frame Disabled {
          n219 = call "W7-X-Bolo-TMDS-LOCAL.vi"("Kappa 2"=w534, "ArrayOutput 4"=w535, "ArrayOutput 3"=w533, "Array"=w532, "RawArray"=w536, "Numeric"=w528, "ArrayOutput"=w529, "Kappa"=w530, "ArrayOutput 2"=w531, "SampleTime"=w527) -> ()  [unwired: 5 in, 1 out]
        }
        frame Enabled {
        }
      }
      n220 = call "Visualize_Signals64.vi"("FPGSampleTime"=w267, "tstart"=w276, "Signals"=w426) -> ("plot(Signals) 33-64"=→"Pow 97 - 128":T26, "plot(Signals) 1-32"=→"Pow 65 - 96":T5)  [unwired: 7 in]
      n221 = call "Visualize_Signals64.vi"("FPGSampleTime"=w267, "tstart"=w276, "Signals"=w430) -> ("plot(Signals) 33-64"=→"Pow 33-64":T26, "plot(Signals) 1-32"=→"Pow 1-32":T5)  [unwired: 7 in]
      n222 = call "Visualize_Signals64.vi"("FPGSampleTime"=w267, "tstart"=w276, "Signals"=w305) -> ("plot(Signals) 33-64"=→"Raw 97 - 128":T26, "plot(Signals) 1-32"=→"Raw 65 - 97":T5)  [unwired: 7 in]
      n223 = call "Visualize_Signals64.vi"("FPGSampleTime"=w267, "tstart"=w276, "Signals"=w300) -> ("plot(Signals) 33-64"=→"Raw 33-64":T26, "plot(Signals) 1-32"=→"Raw 1-32":T5)  [unwired: 7 in]
      n224 = Array Subset(array=w327, index (row)=0 ("index"), length (row)=128 ("length")) -> (w328:dbl[][])  [unwired: 2 in]
      "Fehler READ U+P" <- w291
    }
    frame True {
      n225 = local write "state"("Error->NoRead" ("state")) -> ()
    }
  }
  n226 = xnode "Read/Write Control"("FPGA VI Reference In"=w56) -> ("FPGA VI Reference Out"=w29:refnum<k20>, "SampleTrigger2"=w57:u32)  [unwired: 1 in, 1 out]
  n227 = Multiply(x=w31, y=w30) -> (x*y=w9:i64)
  n228 = To Quad Integer(1:w57) -> (0:w25:i64)
  "Presamples \n(If -1, then no trigger detected)" <- w25
  n229 = flat-sequence {
    tunnel: w59 -> [w730]
    tunnel: w209 -> [w731]
    tunnel: w29 -> [w732]
    tunnel: [w732] -> w28
    tunnel: [w731] -> w27
    tunnel: [w730] -> w26
    tunnel: w9 -> [w729]
    tunnel: w25 -> [w728]
    tunnel: [w727] -> w24
    tunnel: [w745] -> w23
    tunnel: [w744] -> w22
    tunnel: [w743] -> w21
    tunnel: w28 -> [w745]
    tunnel: w27 -> [w744]
    tunnel: w26 -> [w743]
    tunnel: w23 -> [w752]
    tunnel: [w752] -> w19
    tunnel: w22 -> [w751]
    tunnel: [w751] -> w17
    tunnel: w21 -> [w750]
    tunnel: [w750] -> w15
    tunnel: [w748] -> w20
    tunnel: w19 -> [w759]
    tunnel: [w759] -> w18
    tunnel: w17 -> [w758]
    tunnel: [w758] -> w16
    tunnel: w15 -> [w757]
    tunnel: [w757] -> w14
    tunnel: w18 -> [w765]
    tunnel: w16 -> [w763]
    tunnel: w14 -> [w762]
    frame #0 {
      n230 = case "Correct timebase depending on if Trigger detected" shown="4294967295" w728 {
        selector: w728 -> [w735 _]
        tunnel: [w736 w738] -> w727
        tunnel: w729 -> [w734 _]
        frame Default {
          # "1 Trigger nur während OP"
          # "4294967295"
          # "Trigger deviation [ns]"
          # "Input Sample Frequency"
          n231 = Multiply(x=w735, y=w734) -> (x*y=w733:i64)
          n232 = To Quad Integer(1:w733) -> (0:w736:i64)
        }
        frame 4294967295 {
          # "ms to ns conversion"
          # "4294967295\n=default if not Trigger"
          n233 = local read "DAQ wait time (should be = TWT"() -> (w737:i32)
          n234 = Multiply(x=i64 1000000, y=w737) -> (x*y=w738:i64)
        }
      }
    }
    frame #1 {
      n235 = control-ref of="DAQ Timer"() -> (w740:refnum<vi>)
      n236 = call "W7X-Bolo-Timer.vi"("Wait-Time until Trigger\npublished on CODA\ntypically 10 s"="Wait-Time until Trigger\npublished on CODA\ntypically 10 s", "Digital in"=w740) -> ()  [unwired: 10 in]
      n237 = local write "state"("Wait for published Shot Time (10s)" ("state")) -> ()
    }
    frame #2 {
      n238 = case shown="1, Default" "Trigger Source" {
        tunnel: [w753 w755 "Set Manual Time [ns]"] -> w748
        tunnel: "Trigger No Choice\nfrom MDS+ Website\n0 for old\n1 during OP" -> [_ w754 _]
        frame 0 {
          n239 = call "Get UTC from NTP.vi"() -> ("UTC Time"=w753:i64)  [unwired: 10 in, 1 out]
        }
        frame 1, Default {
          n240 = call "GetTriggerTime.vi"("TriggerIndex (1)"=w754) -> ("TriggerTime [ns]"=w755:i64)  [unwired: 9 in, 1 out]
        }
        frame 2 {
        }
      }
      n241 = local write "state"("Reading Trigger Time" ("state")) -> ()
    }
    frame #3 {
    }
    frame #4 {
      n242 = case shown="True" w762 {
        tunnel: w765 -> [w766 w768]
        tunnel: w763 -> [_ w767]
        tunnel: [w766 _] -> w761
        frame False {
        }
        frame True {
          n243 = xnode "Close FPGA VI Reference"("FPGA VI Reference In"=w768, "error in"=w767) -> ()  [unwired: 1 out]
        }
      }
      "FPGA VI Reference Out" <- w761
      n244 = local write "state"("Idle / Waiting for new Trigger" ("state")) -> ()
      n245 = property on="stop" class="Bool (strict)"("Val(Sgnl)"=TRUE) -> ()  [unwired: 2 in, 2 out]
    }
  }
  n246 = call "Array_Trans.vi"("RB01"=w122, "Array 8"=w12, "Kappa 2"=w120, "RB01 2"=w123, "Tau 2"=w121, "Kappa"=w61, "Tau"=w62) -> ("Array 7"=w116:dbl[][], "Array 4"=w111:dbl[][], "Array"=w106:dbl[][], "Array 3"=w109:dbl[][], "Array 6"=w115:dbl[][], "Array 2"=w107:dbl[][], "Array 5"=w113:dbl[][])  [unwired: 2 in]
  n247 = Multiply(x=w9, y=w11) -> (x*y=w10:i64)
  n248 = local read "No. of Samples:"() -> (w13:u32)
  n249 = Add(x=w20, y=w24) -> (x+y=w38:i64)
  n250 = To Quad Integer(1:w38) -> (0:w167:i64)
  n251 = Build Array(w38) -> (w64:i64[])
  n252 = call "W7X2DJSON.vi"("values"=w116, "label"=w90, "dimensionSize"=w36, "dimensions"=w64, "dimensionCount"=128, "sampleCount"=w36, "datatype"=w118) -> ("JSON string"=w89:string)  [unwired: 4 in]
  n253 = call "W7X2DJSON.vi"("values"=w106, "label"=w71, "dimensionSize"=w69, "dimensions"=w64, "dimensionCount"=128, "sampleCount"=w69, "datatype"=w134) -> ("JSON string"=w70:string)  [unwired: 4 in]
  n254 = call "W7X2DJSON.vi"("values"=w115, "label"=w87, "dimensionSize"=w67, "dimensions"=w64, "dimensionCount"=128, "sampleCount"=w67, "datatype"=w124) -> ("JSON string"=w86:string)  [unwired: 4 in]
  n255 = call "W7X2DJSON.vi"("values"=w113, "label"=w84, "dimensionSize"=w112, "dimensions"=w64, "dimensionCount"=128, "sampleCount"=w112, "datatype"=w126) -> ("JSON string"=w83:string)  [unwired: 4 in]
  n256 = Initialize Array(w38, w13) -> (w136:i64[])
  n257 = for {
    N: w13 -> [_]
    shift-right: [w773] -> w54
    shift-left: w136 -> [w774]
    shift-right: [w770] -> _
    shift-left: w38 -> [w771]
    tunnel: w10 -> [w769]
    i -> [w772]
    n258 = Add(x=w771, y=w769) -> (x+y=w770:i64)
    n259 = Replace Array Subset(array=w774, new element=w771, index=w772) -> (w773:i64[])
  }
  n260 = call "W7X2DJSON.vi"("values"=w111, "label"=w81, "dimensionSize"=w110, "dimensions"=w64, "dimensionCount"=128, "sampleCount"=w110, "datatype"=w128) -> ("JSON string"=w80:string)  [unwired: 4 in]
  n261 = call "W7X2DJSON.vi"("values"=w109, "label"=w78, "dimensionSize"=w108, "dimensions"=w64, "dimensionCount"=128, "sampleCount"=w108, "datatype"=w130) -> ("JSON string"=w77:string)  [unwired: 4 in]
  n262 = call "W7X2DJSON.vi"("values"=w107, "label"=w74, "dimensionSize"=w68, "dimensions"=w64, "dimensionCount"=128, "sampleCount"=w68, "datatype"=w132) -> ("JSON string"=w73:string)  [unwired: 4 in]
  n263 = Initialize Array(w20, w37) -> (w135:i64[])
  n264 = for {
    N: w37 -> [_]
    shift-right: [w779] -> w51
    shift-left: w135 -> [w780]
    shift-right: [w776] -> _
    shift-left: w38 -> [w777]
    tunnel: w10 -> [w775]
    i -> [w778]
    n265 = Add(x=w777, y=w775) -> (x+y=w776:i64)
    n266 = Replace Array Subset(array=w780, new element=w777, index=w778) -> (w779:i64[])
  }
  n267 = local read "SampleTime"() -> (w35:sgl)
  n268 = local read "SampleTime"() -> (w2:sgl)
  n269 = Reciprocal(x=w35) -> (1/x=w47:sgl)
  n270 = Reciprocal(x=w35) -> (1/x=w45:sgl)
  n271 = Reciprocal(x=w35) -> (1/x=w43:sgl)
  n272 = Reciprocal(x=w2) -> (1/x=w39:sgl)
  n273 = Reciprocal(x=w2) -> (1/x=w41:sgl)
  n274 = To Unsigned Word Integer(number=w39) -> (unsigned 16bit integer=w4:u16)
  n275 = To Unsigned Word Integer(number=w41) -> (unsigned 16bit integer=w40:u16)
  n276 = call "W7X2DJSON.vi"("values"=w141, "label"=w6, "dimensionSize"=w148, "dimensions"=w51, "dimensionCount"=128, "sampleCount"=w148, "datatype"=w150) -> ("JSON string"=w5:string)  [unwired: 4 in]
  n277 = call "W7X2DJSON.vi"("values"=w138, "label"=w99, "dimensionSize"=w145, "dimensions"=w51, "dimensionCount"=128, "sampleCount"=w145, "datatype"=w147) -> ("JSON string"=w98:string)  [unwired: 4 in]
  n278 = call "W7X2DJSON.vi"("values"=w140, "label"=w95, "dimensionSize"=w151, "dimensions"=w51, "dimensionCount"=128, "sampleCount"=w151, "datatype"=w153) -> ("JSON string"=w94:string)  [unwired: 4 in]
  n279 = call "W7X2DJSON.vi"("values"=w139, "label"=w105, "dimensionSize"=w142, "dimensions"=w51, "dimensionCount"=128, "sampleCount"=w142, "datatype"=w144) -> ("JSON string"=w104:string)  [unwired: 4 in]
  n280 = call "W7X2DJSON.vi"("values"=w154, "label"=w92, "dimensionSize"=w13, "dimensions"=w54, "dimensionCount"=128, "sampleCount"=w13, "datatype"=w155) -> ("JSON string"=w91:string)  [unwired: 4 in]
  n281 = To Unsigned Word Integer(number=w47) -> (unsigned 16bit integer=w46:u16)
  n282 = To Unsigned Word Integer(number=w45) -> (unsigned 16bit integer=w44:u16)
  n283 = To Unsigned Word Integer(number=w43) -> (unsigned 16bit integer=w42:u16)
  n284 = Multiply(x=w13, y=w35) -> (x*y=w34:sgl)
  n285 = Replace Array Subset(array=i64[] [1399090569999999999, -1] ("dimensions"), new element=w167, index=0) -> (w1:i64[])
  n286 = call "W7X1DPut.vi"("dimensions"=w1, "Unit"=w88, "SigJSONbuffer"=w89, "SigLabel"=w90) -> ()  [unwired: 8 in]
  n287 = call "W7X1DPut.vi"("dimensions"=w1, "Unit"=w72, "SigJSONbuffer"=w70, "SigLabel"=w71) -> ()  [unwired: 8 in]
  n288 = call "W7X1DPut.vi"("dimensions"=w1, "Unit"=w85, "SigJSONbuffer"=w86, "SigLabel"=w87) -> ()  [unwired: 8 in]
  n289 = call "W7X1DPut.vi"("dimensions"=w1, "Unit"=w82, "SigJSONbuffer"=w83, "SigLabel"=w84) -> ()  [unwired: 8 in]
  n290 = call "W7X1DPut.vi"("dimensions"=w1, "Unit"=w79, "SigJSONbuffer"=w80, "SigLabel"=w81) -> ()  [unwired: 8 in]
  n291 = call "W7X1DPut.vi"("dimensions"=w1, "Unit"=w76, "SigJSONbuffer"=w77, "SigLabel"=w78) -> ()  [unwired: 8 in]
  n292 = call "W7X1DPut.vi"("dimensions"=w1, "Unit"=w75, "SigJSONbuffer"=w73, "SigLabel"=w74) -> ()  [unwired: 8 in]
  n293 = call "W7X2DPut.vi"("dimensions"=w1, "pulse_length"=w34, "Unit"=w93, "sample period"=w35, "sample rate"=w42, "SigJSONbuffer"=w91, "SigLabel"=w92) -> ()  [unwired: 4 in, 1 out]
  n294 = call "W7X2DPut.vi"("dimensions"=w1, "pulse_length"=4.0, "Unit"=w97, "sample period"=w35, "sample rate"=w46, "SigJSONbuffer"=w94, "SigLabel"=w95) -> ()  [unwired: 4 in, 1 out]
  n295 = call "W7X2DPut.vi"("dimensions"=w1, "pulse_length"=4.0, "Unit"=w103, "sample period"=w2, "sample rate"=w44, "SigJSONbuffer"=w104, "SigLabel"=w105) -> ("Parlog error out"=→"Parlog error out":errorcluster)  [unwired: 4 in]
  n296 = call "W7X2DPut.vi"("dimensions"=w1, "pulse_length"=4.0, "Unit"=w101, "sample period"=w2, "sample rate"=w40, "SigJSONbuffer"=w98, "SigLabel"=w99) -> ("Parlog error out"=→"Parlog error out  2":errorcluster)  [unwired: 4 in]
  n297 = call "W7X2DPut_DAZ.vi"("dimensions"=w1, "pulse_length"=4.0, "Unit"=w7, "sample period"=w2, "sample rate"=w4, "SigJSONbuffer"=w5, "SigLabel"=w6) -> ()  [unwired: 4 in, 1 out]
  n298 = call "chanDescQSB.vi"("dimensions"=w1, "values"=T19 [{"chanDescs"=[{"name"="E_Chan_1", "active"=1}, {"name"="E_Chan_2", "active"=1}, {"name"="E_Chan_3", "active"=1}, {"name"="E_Chan_4", "active"=1}, {"name"="E_Chan_5", "active"=1}, {"name"="E_Chan_6", "active"=1}, {"name"="E_Chan_7", "active"=1}, {"name"="E_Chan_8", "active"=1}, {"name"="E_Chan_9", "active"=1}, {"name"="E_Chan_10", "active"=1}, {"name"="E_Chan_11", "active"=1}, {"name"="E_Chan_12", "active"=1}, {"name"="E_Chan_13", "active"=1}, {"name"="E_Chan_14", "active"=1}, {"name"="E_Chan_15", "active"=1}, {"name"="E_Chan_16", "active"=1}, {"name"="E_Chan_17", "active"=1}, {"name"="E_Chan_18", "active"=1}, {"name"="E_Chan_19", "active"=1}, {"name"="E_Chan_20", "active"=1}, {"name"="E_Chan_21", "active"=1}, {"name"="E_Chan_22", "active"=1}, {"name"="E_Chan_23", "active"=1}, {"name"="E_Chan_24", "active"=1}, {"name"="E_Chan_25", "active"=1}, {"name"="E_Chan_26", "active"=1}, {"name"="E_Chan_27", "active"=1}, {"name"="E_Chan_28", "active"=1}, {"name"="E_Chan_29", "active"=1}, {"name"="E_Chan_30", "active"=1}, {"name"="E_Chan_31", "active"=1}, {"name"="E_Chan_32", "active"=1}, {"name"="E_Chan_33", "active"=1}, {"name"="E_Chan_34", "active"=1}, {"name"="E_Chan_35", "active"=1}, {"name"="E_Chan_36", "active"=1}, {"name"="E_Chan_37", "active"=1}, {"name"="E_Chan_38", "active"=1}, {"name"="E_Chan_39", "active"=1}, {"name"="E_Chan_40", "active"=1}, {"name"="E_Chan_41", "active"=1}, {"name"="E_Chan_42", "active"=1}, {"name"="E_Chan_43", "active"=1}, {"name"="E_Chan_44", "active"=1}, {"name"="E_Chan_45", "active"=1}, {"name"="E_Chan_46", "active"=1}, {"name"="E_Chan_47", "active"=1}, {"name"="E_Chan_48", "active"=1}, {"name"="E_Chan_49", "active"=1}, {"name"="E_Chan_50", "active"=1}, {"name"="E_Chan_51", "active"=1}, {"name"="E_Chan_52", "active"=1}, {"name"="E_Chan_53", "active"=1}, {"name"="E_Chan_54", "active"=1}, {"name"="E_Chan_55", "active"=1}, {"name"="E_Chan_56", "active"=1}, {"name"="E_Chan_57", "active"=1}, {"name"="E_Chan_58", "active"=1}, {"name"="E_Chan_59", "active"=1}, {"name"="E_Chan_60", "active"=1}, {"name"="E_Chan_61", "active"=1}, {"name"="E_Chan_62", "active"=1}, {"name"="E_Chan_63", "active"=1}, {"name"="E_Chan_64", "active"=1}, {"name"="E_Chan_65", "active"=1}, {"name"="E_Chan_66", "active"=1}, {"name"="E_Chan_67", "active"=1}, {"name"="E_Chan_68", "active"=1}, {"name"="E_Chan_69", "active"=1}, {"name"="E_Chan_70", "active"=1}, {"name"="E_Chan_71", "active"=1}, {"name"="E_Chan_72", "active"=1}, {"name"="E_Chan_73", "active"=1}, {"name"="E_Chan_74", "active"=1}, {"name"="E_Chan_75", "active"=1}, {"name"="E_Chan_76", "active"=1}, {"name"="E_Chan_77", "active"=1}, {"name"="E_Chan_78", "active"=1}, {"name"="E_Chan_79", "active"=1}, {"name"="E_Chan_80", "active"=1}, {"name"="E_Chan_81", "active"=1}, {"name"="E_Chan_82", "active"=1}, {"name"="E_Chan_83", "active"=1}, {"name"="E_Chan_84", "active"=1}, {"name"="E_Chan_85", "active"=1}, {"name"="E_Chan_86", "active"=1}, {"name"="E_Chan_87", "active"=1}, {"name"="E_Chan_88", "active"=1}, {"name"="E_Chan_89", "active"=1}, {"name"="E_Chan_90", "active"=1}, {"name"="E_Chan_91", "active"=1}, {"name"="E_Chan_92", "active"=1}, {"name"="E_Chan_93", "active"=1}, {"name"="E_Chan_94", "active"=1}, {"name"="E_Chan_95", "active"=1}, {"name"="E_Chan_96", "active"=1}, {"name"="E_Chan_97", "active"=1}, {"name"="E_Chan_98", "active"=1}, {"name"="E_Chan_99", "active"=1}, {"name"="E_Chan_100", "active"=1}, {"name"="E_Chan_101", "active"=1}, {"name"="E_Chan_102", "active"=1}, {"name"="E_Chan_103", "active"=1}, {"name"="E_Chan_104", "active"=1}, {"name"="E_Chan_105", "active"=1}, {"name"="E_Chan_106", "active"=1}, {"name"="E_Chan_107", "active"=1}, {"name"="E_Chan_108", "active"=1}, {"name"="E_Chan_109", "active"=1}, {"name"="E_Chan_110", "active"=1}, {"name"="E_Chan_111", "active"=1}, {"name"="E_Chan_112", "active"=1}, {"name"="E_Chan_113", "active"=1}, {"name"="E_Chan_114", "active"=1}, {"name"="E_Chan_115", "active"=1}, {"name"="E_Chan_116", "active"=1}, {"name"="E_Chan_117", "active"=1}, {"name"="E_Chan_118", "active"=1}, {"name"="E_Chan_119", "active"=1}, {"name"="E_Chan_120", "active"=1}, {"name"="E_Chan_121", "active"=1}, {"name"="E_Chan_122", "active"=1}, {"name"="E_Chan_123", "active"=1}, {"name"="E_Chan_124", "active"=1}, {"name"="E_Chan_125", "active"=1}, {"name"="E_Chan_126", "active"=1}, {"name"="E_Chan_127", "active"=1}, {"name"="E_Chan_128", "active"=1}]}], "label"="parms") -> ()  [unwired: 1 out]
  n299 = call "parmsQSB.vi"("dimensions"=w1, "values"=T18 [{"Nchannel"=128, "ADCbits"=16, "BridgeVoltage (V)"=5.0, "ExptSampleFrequency (Hz)"=2500.0, "CalibSampleFrequency (Hz)"=2500.0, "CalStep1 (V)"="2.5", "CalStep2 (V)"="3.7", "detector"="Au_Kapton"}], "label"="parms") -> ("JSON string"=w53:string)
  n300 = call <vilib>:"OpenHandle.vi"() -> ("client handle out"=w164:T29, "error out"=w163:errorcluster)  [unwired: 14 in]
  n301 = call <vilib>:"AddHeader.vi"("client handle"=w164, "header"="Content-Type", "value"="application/json", "error in (no error)"=w163) -> ("client handle out"=w162:T29, "error out"=w161:errorcluster)  [unwired: 10 in]
  n302 = call-poly <vilib>:"POST.vi"("client handle"=w162, "url"="http://archive-webapi/Test/raw/W7X/QSB_Bolometry/File_PARLOG/", "buffer"=w53, "error in (no error)"=w161, "timeout (10000)"=400000 ("timeout for upload")) -> ("client handle out"=w166:T29, "headers"=→"headers chanDesc":string, "body"=→"body chanDesc":string, "error out"=w48:errorcluster)  [unwired: 7 in]
  n303 = call <vilib>:"CloseHandle.vi"("client handle"=w166, "error in (no error)"=w48) -> ("error out"=w156:errorcluster)  [unwired: 13 in]
  n304 = call "saveToFile.vi"("SigJSONbuffer"=w53, "dimensions"=w51, "String"="File_PARLOG" ("name or relative path")) -> ("error out"=w49:errorcluster)  [unwired: 8 in]
  n305 = Merge Errors(w156, w49) -> (→"parms error out":errorcluster)
